vi "ME_acquire_22_HallSensor_LSchanB.vi"() -> ()   [LabVIEW 2015]
doc: "Use this template to build a producer/consumer design pattern. Use this template when you need to execute a process, such as data analysis, when a data source, such as a triggered acquisition, produces data at an uneven rate and you need to execute the process when the data becomes available."
uses:
  Mode.ctl
  oxford_driver/Oxford Drivers/BUSGEN.LLB/OxfordAddress.ctl
  <vilib>/Analysis/baseanly.llb/Mean (DBL).vi
  <vilib>/DAQmx/read.llb/DAQmx Read (Analog 1D DBL 1Chan NSamp).vi
  <vilib>/DAQmx/create/channels.llb/DAQmx Create Channel (AI-Voltage-Basic).vi
  <vilib>/DAQmx/configure/timing.llb/DAQmx Timing (Sample Clock).vi
  <vilib>/Utility/file.llb/Write Delimited Spreadsheet (DBL).vi
  <vilib>/DAQmx/miscellaneous.llb/DAQmx Fill In Error Info.vi
  <vilib>/express/express arith-compare/Formula/XNode/ExpressFormulaBlockNode.xnode
  <vilib>/Analysis/NI_AALBase.lvlib
panel:
  out "error out 2":errorcluster
  out "concatenated string":string
  out "error out":errorcluster
  out "B lag":cluster{dbl[], dbl[]}(graph)
  out "T array":dbl[](array[numeric])
  out "Averaged I(T)":dbl[][](array[numeric])
  in  "Averaged P(T)":dbl[][](array[numeric])
  out "remaining elements 2":T1(array[cluster])
  out "Actual mean":dbl format="%0.6f"
  in  "Averaged dt":dbl[][](array[numeric])
  in  "Averaged P(B)":dbl[][](array[numeric])
  out "deltaUaux":dbl
  out "Hall Resistance (Ohm)":dbl caption="Actual AuxV" step=0.1
  in  "Stop":bool
  out "SaveSweep":bool=TRUE
  out "Measurement File_dn":path
  out "Measurement File_up":path
  out "Measurement File_average":path
  out "Actual Polarization":dbl
  in  "Reset IB?":bool
  in  "First?":bool
  in  "Save Period":dbl=1.0
  out "Averaged I(B)":dbl[][](array[numeric])
  out "P(uC/mm^2)":dbl[](array[numeric])
  in  "Sweep":bool
  out "Offset array":dbl[](array[numeric])
  in  "stop 2":bool
  in  "dB":dbl=0.005
  out "Actual B Field (T)":dbl
  out "Actual Temperature (K)":dbl
  out "Actual Current (pA)":dbl
  in  "Tab Control":T2(tab)
  in  "Heater 2/1":bool
  in  "dt (K)":dbl=0.1
  in  "Max temperature (K)":dbl=20.0
  in  "Min Temperature (K)":dbl=4.5
  out "P(T)":cluster{"yi":dbl[], dbl[]}(graph)
  out "I(T)":cluster{dbl[], dbl[]}(graph)
  in  "Set temperature (K)":dbl=4.5
  in  "Temp Ramping Rate (K/min)":dbl=10.0
  in  "Heater Range":enum16{"Off", "Low", "Medium", "High"}(ring)
  in  "Heater On/Off":bool
  out "Setpoint Temperature (K)":dbl
  out "I(T) /Averaged/":cluster{"B array":dbl[], dbl[]}[](graph)
  out "P(T) /Averaged/":cluster{"B array":dbl[], dbl[]}[](graph)
  out "Up/Down 2":bool
  in  "Channel B/A":bool
  out "I(B) 3":cluster{dbl[], dbl[]}[](graph)
  out "I(B) /Averaged/":cluster{"B array":dbl[], dbl[]}[](graph)
  out "P(B) /Averaged/":cluster{"B array":dbl[], dbl[]}[](graph)
  out "P(B)":cluster{"yi":dbl[], dbl[]}(graph)
  in  "Set Field (T)":dbl
  in  "Go to Set":bool
  in  "Sweep Rate (T/min)":dbl=2.0 format="%.6f"
  in  "Field To Zero":bool
  out "Target Field":dbl
  in  "Min Field (T)":dbl
  in  "Max Field (T)":dbl=0.15
  in  "Threshold B (T)":dbl
  out "Up/Down":bool
  in  "Heater Range Array":i8[](array[numeric])=[1, 1, 1, 1, 1, 2, 2, 2, 2]
  in  "Magnetic Field array (T)":dbl[](array[numeric])=[0.025, 0.05, 0.075, 0.1, 0.125, 0.15, 0.175, 0.2, 0.225, 0.25, 0.275, 0.3]
  in  "T Sweep Rate Array":dbl[](array[numeric])=[10.0, 20.0]
  in  "Max count array":i32[](array[numeric])=[2, 1, 0, 0, 0, 9, 10, 11, 12]
  in  "secs to wait":dbl=180.0
  out "Wait (s)":dbl
  in  "Directory":string
  out "Finished":bool=TRUE
  out "Step Rate":bool
  out "New":bool=TRUE
  in  "Temperature Array":dbl[](array[numeric])=[4.5, 5.0, 6.0, 7.0, 8.0, 9.0, 10.0, 11.0, 12.0]
  in  "Sweep Rate Array":dbl[](array[numeric])=[2.0, 1.0, 0.5, 0.1, 0.05, 9.0, 10.0, 11.0, 12.0]
  in  "Record ALL":bool
  in  "Max Countl":i32
  out "i":i32
  out "j":i32
  out "Step Temp":bool
  in  "FileName":string
  in  "Measure Noise":bool
  in  "Cycles":i32
  in  "maximum value":dbl=10.0 format="%0.2f"
  in  "minimum value":dbl=-10.0 format="%0.2f"
  in  "physical channels":tag="Dev1/ai1"
  out "PSD (pA/Hz^1/2) Peaks Removed":cluster{"f0":dbl, "df":dbl, "magnitude":dbl[]}(graph)
  out "PSD (pA/Hz^1/2)":cluster{"f0":dbl, "df":dbl, "magnitude":dbl[]}(graph)
  out "Current (pA) Filtered":waveform(dbl)(graph)
  out "Current (pA)":dbl[](graph)
  in  "Samples per channel":i32=1000
  in  "Rate":dbl=1000.0 format="%0.2f"
  in  "Cut-Off Frequency":dbl=100.0 caption="Lower Cut-Off"
  in  "Filter On":bool
  in  "Keithley (IV conv) averaging":i32=10
  in  "Lock_in_Amplifier":refnum<visa-resource-name>="GPIB0::5::INSTR"
  out "Dc offset":dbl
  in  "Calibrate":bool
  in  "IV converter":refnum<visa-resource-name>="GPIB0::20::INSTR"
  in  "Magnetic Field":refnum<visa-resource-name>="GPIB0::19::INSTR"
  out "Time Lag":dbl=0.0500025749206543
  in  "Lake Shore":refnum<visa-resource-name>="GPIB0::11::INSTR"
  in  "Temp Refresh (s)":dbl=0.1
  in  "Sampling rate (Hz)":dbl=10.0
  in  "Gain (V/A)":dbl=1000000000.0
  in  "Sample area (mm^2)":dbl=1.0
  out "Calibration Curve":cluster{dbl[], "Best Linear Fit":dbl[]}[](graph)=[{[0.0, 0.005, 0.01, 0.015, 0.02, 0.025, 0.03, 0.035, 0.04, 0.045, 0.05, 0.055, 0.06, 0.065, 0.07, 0.075, 0.08, 0.085, 0.09, 0.095, 0.1, 0.105, 0.11, 0.115, 0.12, 0.125, 0.13, 0.135, 0.14, 0.145, 0.15, 0.155, 0.16, 0.165, 0.17, 0.175, 0.18, 0.185, 0.19, 0.195, 0.2, 0.205, 0.21, 0.215, 0.22, 0.225, 0.23, 0.235, 0.24, 0.245, 0.25, 0.255, 0.26, 0.265, 0.27, 0.275, 0.28, 0.285, 0.29, 0.295, 0.3, 0.305, 0.31, 0.315, 0.32, 0.325, 0.33, 0.335, 0.34, 0.345, 0.35, 0.355, 0.36, 0.365, 0.37, 0.375, 0.38, 0.385, 0.39, 0.395, 0.4, 0.405, 0.41, 0.415, 0.42, 0.425, 0.43, 0.435, 0.44, 0.445, 0.45, 0.455, 0.46, 0.465, 0.47, 0.475, 0.48, 0.485, 0.49, 0.495, 0.5], "Best Linear Fit"=[-1.7e-06, 1.18e-05, 3.66e-05, 6.17e-05, 9.39e-05, 0.000122, 0.0001511, 0.0001781, 0.0002061, 0.0002355, 0.0002616, 0.0002895, 0.0003184, 0.0003446, 0.0003689, 0.0003958, 0.0004207, 0.0004464, 0.0004684, 0.0004953, 0.0005218, 0.0005459, 0.0005692, 0.0005897, 0.0006131, 0.0006347, 0.0006589, 0.0006834, 0.0007035, 0.0007249, 0.0007465, 0.000765, 0.0007858, 0.0008103, 0.0008302, 0.0008467, 0.000868, 0.0008855, 0.0009079, 0.0009248, 0.0009452, 0.0009633, 0.0009828, 0.0009992, 0.0010189, 0.0010338, 0.001054, 0.0010692, 0.0010858, 0.0011036, 0.0011162, 0.0011356, 0.0011502, 0.0011643, 0.0011834, 0.0011985, 0.0012131, 0.0012277, 0.0012423, 0.0012571, 0.0012691, 0.0012827, 0.0012976, 0.001313, 0.0013264, 0.0013388, 0.0013518, 0.0013638, 0.0013782, 0.0013909, 0.0014035, 0.0014175, 0.0014295, 0.0014407, 0.0014538, 0.0014641, 0.0014752, 0.0014861, 0.0014978, 0.0015081, 0.0015203, 0.001532, 0.0015422, 0.0015526, 0.001563, 0.0015754, 0.0015844, 0.0015955, 0.0016056, 0.001614, 0.0016239, 0.0016342, 0.0016457, 0.0016542, 0.0016635, 0.001674, 0.001681, 0.0016886, 0.0016986, 0.0017063, 0.0017155]}, {[0.0, 0.005, 0.01, 0.015, 0.02, 0.025, 0.03, 0.035, 0.04, 0.045, 0.05, 0.055, 0.06, 0.065, 0.07, 0.075, 0.08, 0.085, 0.09, 0.095, 0.1, 0.105, 0.11, 0.115, 0.12, 0.125, 0.13, 0.135, 0.14, 0.145, 0.15, 0.155, 0.16, 0.165, 0.17, 0.175, 0.18, 0.185, 0.19, 0.195, 0.2, 0.205, 0.21, 0.215, 0.22, 0.225, 0.23, 0.235, 0.24, 0.245, 0.25, 0.255, 0.26, 0.265, 0.27, 0.275, 0.28, 0.285, 0.29, 0.295, 0.3, 0.305, 0.31, 0.315, 0.32, 0.325, 0.33, 0.335, 0.34, 0.345, 0.35, 0.355, 0.36, 0.365, 0.37, 0.375, 0.38, 0.385, 0.39, 0.395, 0.4, 0.405, 0.41, 0.415, 0.42, 0.425, 0.43, 0.435, 0.44, 0.445, 0.45, 0.455, 0.46, 0.465, 0.47, 0.475, 0.48, 0.485, 0.49, 0.495, 0.5], "Best Linear Fit"=[-1.7e-06, 1.18e-05, 3.66e-05, 6.17e-05, 9.39e-05, 0.000122, 0.0001511, 0.0001781, 0.0002061, 0.0002355, 0.0002616, 0.0002895, 0.0003184, 0.0003446, 0.0003689, 0.0003958, 0.0004207, 0.0004464, 0.0004684, 0.0004953, 0.0005218, 0.0005459, 0.0005692, 0.0005897, 0.0006131, 0.0006347, 0.0006589, 0.0006834, 0.0007035, 0.0007249, 0.0007465, 0.000765, 0.0007858, 0.0008103, 0.0008302, 0.0008467, 0.000868, 0.0008855, 0.0009079, 0.0009248, 0.0009452, 0.0009633, 0.0009828, 0.0009992, 0.0010189, 0.0010338, 0.001054, 0.0010692, 0.0010858, 0.0011036, 0.0011162, 0.0011356, 0.0011502, 0.0011643, 0.0011834, 0.0011985, 0.0012131, 0.0012277, 0.0012423, 0.0012571, 0.0012691, 0.0012827, 0.0012976, 0.001313, 0.0013264, 0.0013388, 0.0013518, 0.0013638, 0.0013782, 0.0013909, 0.0014035, 0.0014175, 0.0014295, 0.0014407, 0.0014538, 0.0014641, 0.0014752, 0.0014861, 0.0014978, 0.0015081, 0.0015203, 0.001532, 0.0015422, 0.0015526, 0.001563, 0.0015754, 0.0015844, 0.0015955, 0.0016056, 0.001614, 0.0016239, 0.0016342, 0.0016457, 0.0016542, 0.0016635, 0.001674, 0.001681, 0.0016886, 0.0016986, 0.0017063, 0.0017155]}]
  in  "Offset?":bool
  in  "Magnet":bool=TRUE
  in  "Ramp":bool=TRUE
  in  "DaQ":bool
  in  "Moving average":i8=10
  in  "Sample Rate":dbl=1000.0
  in  "Number of Samples":i32=100
  in  "Physical Channel":tag="kartya/ai0"
  in  "Min Voltage":dbl=-5.0
  in  "Max Voltage":dbl=5.0
  in  "Terminal Configuration":i32(ring)=-1 items=["default"=-1, "RSE"=10083, "NRSE"=10078, "Differential"=10106, "Pseudodifferential"=12529]
  out "Confirm":bool
  in  "Dwell Time (ms)":u32=1000
  out "Calibration Curve Data":dbl[][](array[numeric])=[[0.0, 0.005, 0.01, 0.015, 0.02, 0.025, 0.03, 0.035, 0.04, 0.045, 0.05, 0.055, 0.06, 0.065, 0.07, 0.075, 0.08, 0.085, 0.09, 0.095, 0.1, 0.105, 0.11, 0.115, 0.12, 0.125, 0.13, 0.135, 0.14, 0.145, 0.15, 0.155, 0.16, 0.165, 0.17, 0.175, 0.18, 0.185, 0.19, 0.195, 0.2, 0.205, 0.21, 0.215, 0.22, 0.225, 0.23, 0.235, 0.24, 0.245, 0.25, 0.255, 0.26, 0.265, 0.27, 0.275, 0.28, 0.285, 0.29, 0.295, 0.3, 0.305, 0.31, 0.315, 0.32, 0.325, 0.33, 0.335, 0.34, 0.345, 0.35, 0.355, 0.36, 0.365, 0.37, 0.375, 0.38, 0.385, 0.39, 0.395, 0.4, 0.405, 0.41, 0.415, 0.42, 0.425, 0.43, 0.435, 0.44, 0.445, 0.45, 0.455, 0.46, 0.465, 0.47, 0.475, 0.48, 0.485, 0.49, 0.495, 0.5], [-1.7e-06, 1.18e-05, 3.66e-05, 6.17e-05, 9.39e-05, 0.000122, 0.0001511, 0.0001781, 0.0002061, 0.0002355, 0.0002616, 0.0002895, 0.0003184, 0.0003446, 0.0003689, 0.0003958, 0.0004207, 0.0004464, 0.0004684, 0.0004953, 0.0005218, 0.0005459, 0.0005692, 0.0005897, 0.0006131, 0.0006347, 0.0006589, 0.0006834, 0.0007035, 0.0007249, 0.0007465, 0.000765, 0.0007858, 0.0008103, 0.0008302, 0.0008467, 0.000868, 0.0008855, 0.0009079, 0.0009248, 0.0009452, 0.0009633, 0.0009828, 0.0009992, 0.0010189, 0.0010338, 0.001054, 0.0010692, 0.0010858, 0.0011036, 0.0011162, 0.0011356, 0.0011502, 0.0011643, 0.0011834, 0.0011985, 0.0012131, 0.0012277, 0.0012423, 0.0012571, 0.0012691, 0.0012827, 0.0012976, 0.001313, 0.0013264, 0.0013388, 0.0013518, 0.0013638, 0.0013782, 0.0013909, 0.0014035, 0.0014175, 0.0014295, 0.0014407, 0.0014538, 0.0014641, 0.0014752, 0.0014861, 0.0014978, 0.0015081, 0.0015203, 0.001532, 0.0015422, 0.0015526, 0.001563, 0.0015754, 0.0015844, 0.0015955, 0.0016056, 0.001614, 0.0016239, 0.0016342, 0.0016457, 0.0016542, 0.0016635, 0.001674, 0.001681, 0.0016886, 0.0016986, 0.0017063, 0.0017155]]
  in  "Start Field":dbl
  in  "Max Field":dbl=0.5 format="%#_13g"
  in  "Reoffset?":bool
  in  "Temp/Magnetic Field":bool
  out "index":i8
  out "Read?":bool
  out "Magnetic Field (T)":dbl[](array[numeric])
  out "Reset":bool
  out "Measured Current (pA)":dbl[](array[numeric])
  out "Elapsed Time (s)":dbl[](array[numeric])
  out "Start time":timestamp
  in  "Enum":T3=enum."Process"
  out "B array":dbl[](array[numeric])
  in  "dB (T)":dbl=0.0025
  in  "Counter":i8
  out "L magnet (H)":dbl
  out "R magnet (mOhm)":dbl
  out "Actual Current (R0)":dbl
  out "Nominal Field (T)":dbl
  out "Temperature array":dbl[](array[numeric])
  in  "New Measurement File":bool
  out "Measurement File":path
  out "refnum out":refnum<file>
  in  "Measuring":bool
  in  "Measure /Pause":bool
  in  "stop":bool
  # "DeltaForce"
  # "Discrete"
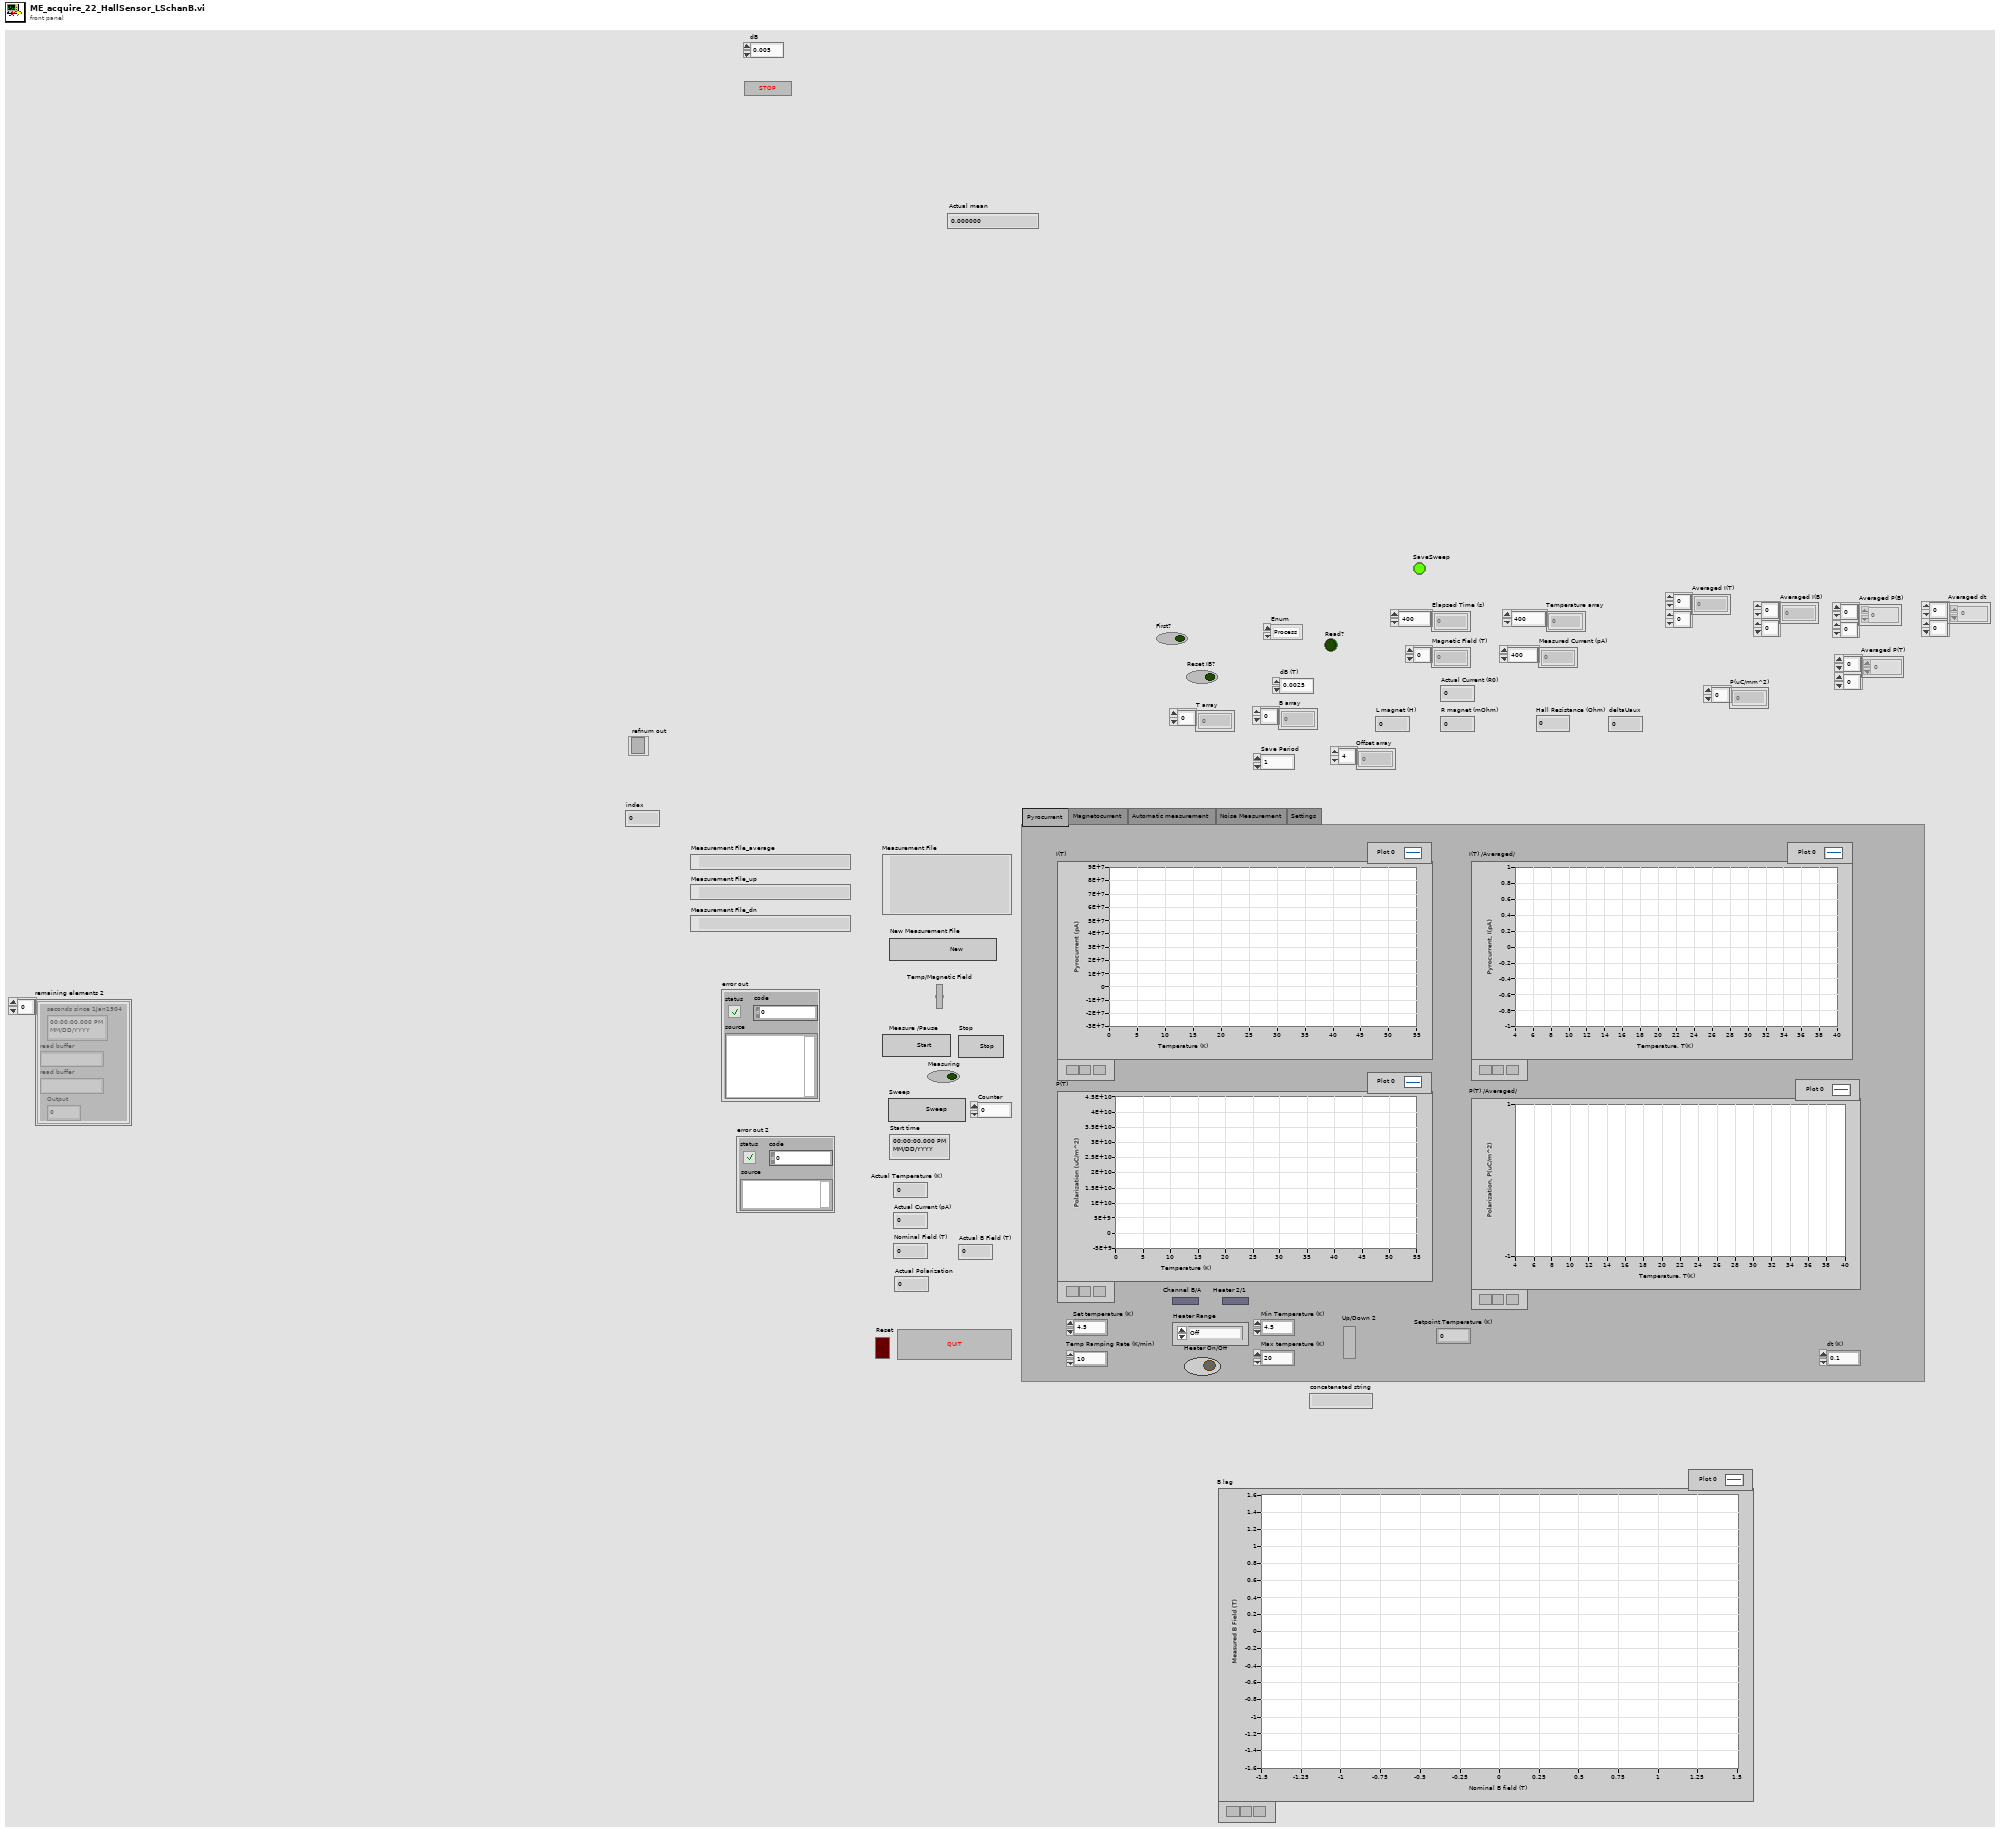
[diagram p1: front panel]
types:
  T1 = cluster{"seconds since 1Jan1904":timestamp, "read buffer":string, "read buffer":string, "Output":dbl}[]
  T2 = enum32{"Pyrocurrent", "Magnetocurrent", "Automatic measurement", "Noise Measurement", "Settings"}
  T3 = typedef "Mode.ctl" = enum16{"Offset", "Process", "Sweep", "StepOxford", "StepDelta", "Plot", "Save", "New", "Return", ""}
  T4 = cluster{"seconds since 1Jan1904":timestamp, "read buffer":string, "read buffer":string, "Output":dbl}
  T5 = enum16{"open", "replace", "create", "open or create", "replace or create", "replace or create with confirmation"}
  T6 = typedef "OxfordAddress.ctl" = cluster{"Com Port":i32, "ISOBUS Address":i32, "GPIB Address":i16, "Communication":enum16{"RS232", "ISOBUS", "GPIB", "Gateway"}}
  T7 = cluster{"B array":dbl[], "Averaged P(B) Out":dbl[]}
  T8 = cluster{"B array":dbl[], "BaselineSubtracted I(B)":dbl[]}
  T9 = cluster{"B array":dbl[], "Averaged P(B) Out":dbl[]}[]
  T10 = cluster{"B array":dbl[], "BaselineSubtracted I(B)":dbl[]}[]
  T11 = cluster{"T array":dbl[], "Averaged P(T) Out":dbl[]}
  T12 = cluster{"T array":dbl[], "Averaged I(B) out":dbl[]}
  T13 = cluster{"T array":dbl[], "Averaged P(T) Out":dbl[]}[]
  T14 = cluster{"T array":dbl[], "Averaged I(B) out":dbl[]}[]
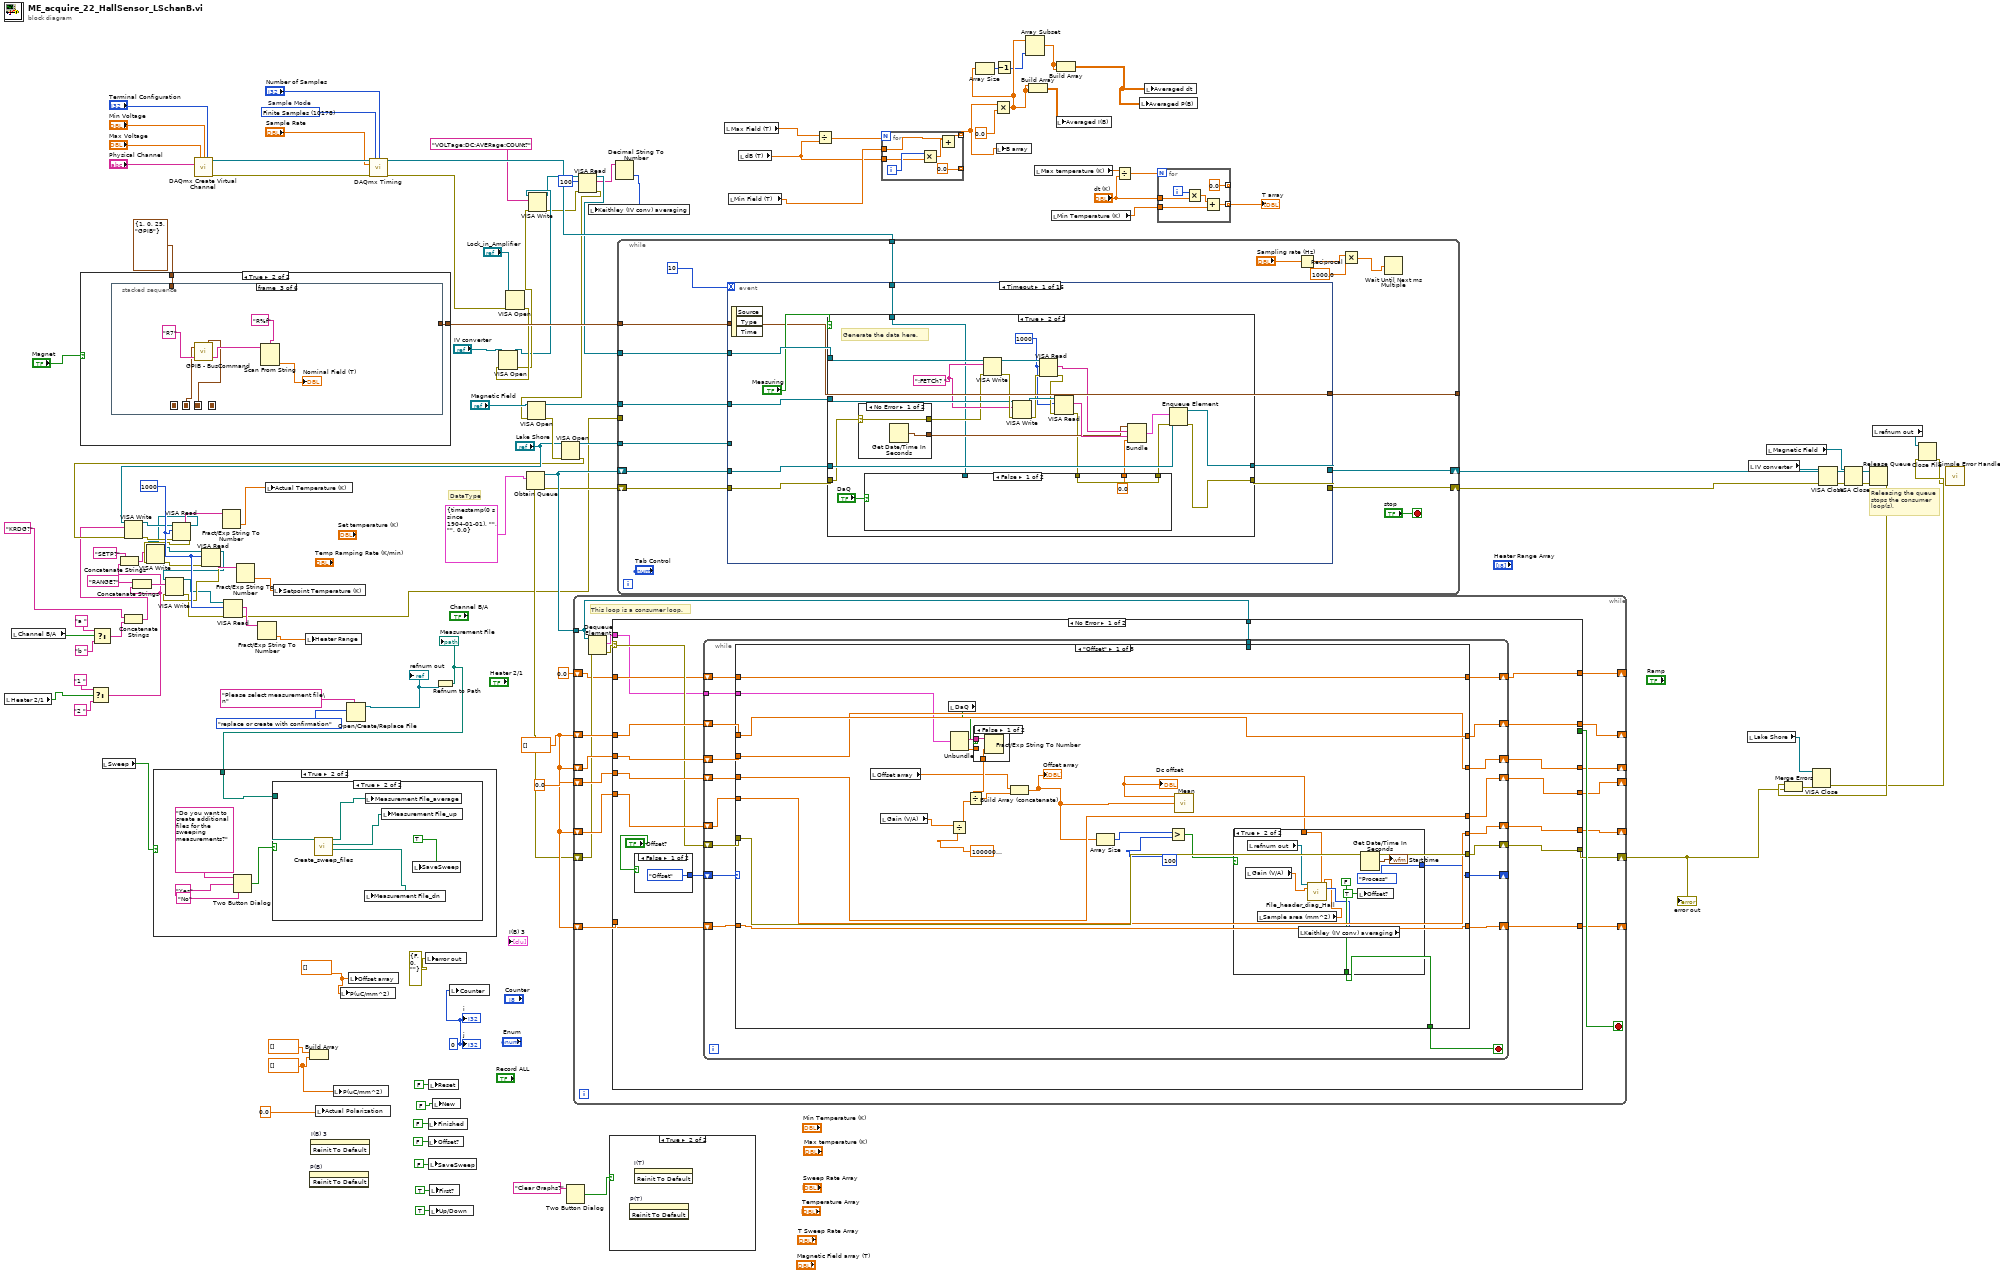
[diagram p0: block diagram]
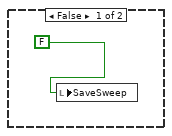
[diagram p4: hidden frame]
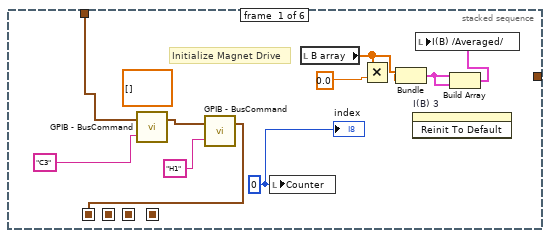
[diagram p6: hidden frame]
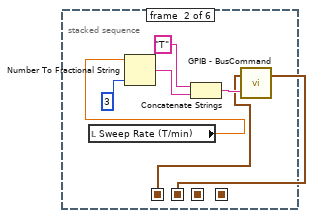
[diagram p7: hidden frame]
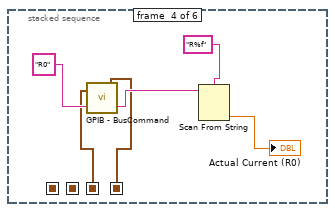
[diagram p8: hidden frame]
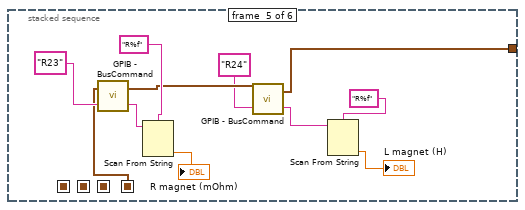
[diagram p9: hidden frame]
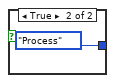
[diagram p11: hidden frame]
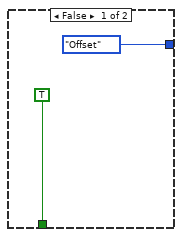
[diagram p13: hidden frame]
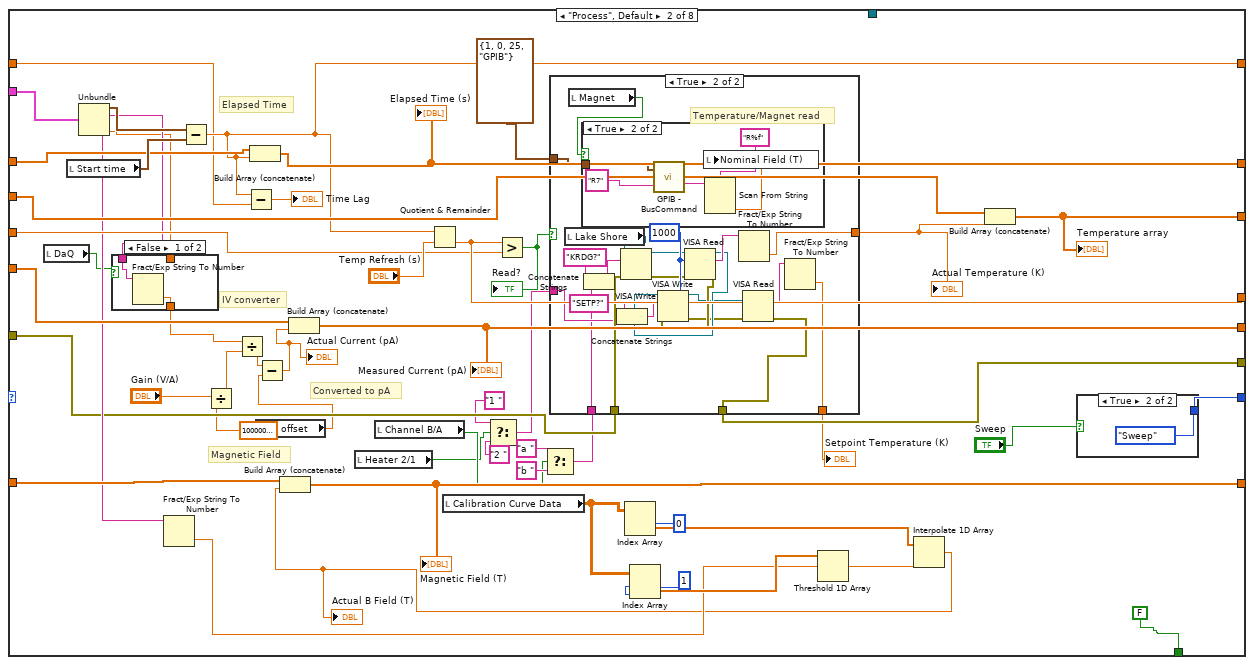
[diagram p14: hidden frame]
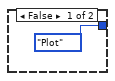
[diagram p16: hidden frame]
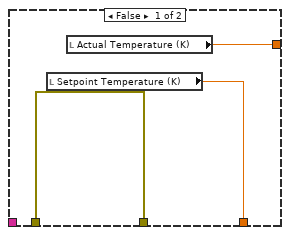
[diagram p17: hidden frame]
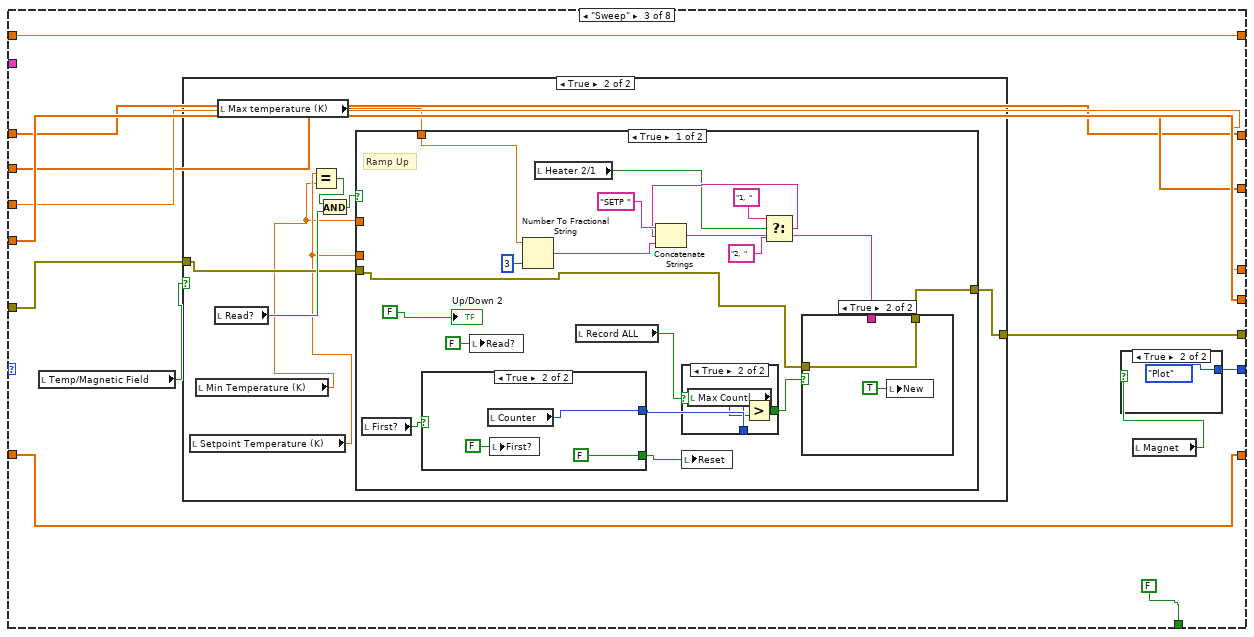
[diagram p19: hidden frame]
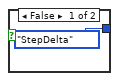
[diagram p20: hidden frame]
diagram:
  w43 = 10178 items=["Finite Samples"=10178, "Continuous Samples"=10123, "Hardware Timed Single Point"=12522]  # Sample Mode
  w70 = u32 1000 ("byte count")
  w78 = 0 ("j")
  w75 = dbl[] []
  w93 = dbl[] []
  w99 = dbl[] []
  # "DataType"
  # "Releasing the queue stops the consumer loop(s)."
  n1 = local read "Heater 2/1"() -> (w1:bool)
  n2 = local read "Channel B/A"() -> (w3:bool)
  n3 = case shown="True" "Magnet" {
    tunnel: T6 {"Com Port"=1, "ISOBUS Address"=0, "GPIB Address"=25, "Communication"=enum."GPIB"} ("Address") -> [w122 w124]
    tunnel: [w122 w123] -> w105
    frame False {
    }
    frame True {
      n4 = stacked-sequence {
        seq-local: [w132 _ _ _ _ _] -> [_ w137 _ _ _ _]
        seq-local: [_ w136 _ _ _ _] -> [_ _ w144 _ _ _]
        seq-local: [_ _ w143 _ _ _] -> [_ _ _ w150 _ _]
        seq-local: [_ _ _ w149 _ _] -> [_ _ _ _ w161 _]
        tunnel: w124 -> [w134 _ _ _ _ _]
        tunnel: [_ _ _ _ w159 _] -> w123
        frame #0 {
          (unwired) dbl[][] []
          w130 = i8 0 ("Counter")
          # "Initialize Magnet Drive"
          n5 = call "GPIB - BusCommand.vi"("Command"="C3", "Address"=w134) -> ("Address(thru)"=w133:T6)  [unwired: 1 out]
          n6 = call "GPIB - BusCommand.vi"("Command"="H1", "Address"=w133) -> ("Address(thru)"=w132:T6)  [unwired: 1 out]
          n7 = local write "Counter"(w130) -> ()
          n8 = local read "B array"() -> (w128:dbl[])
          n9 = Multiply(x=w128, y=0.0) -> (x*y=w127:dbl[])
          n10 = Bundle("B array"=w128, w127) -> (w126:cluster{"B array":dbl[], dbl[]})  [unwired: 1 in]
          n11 = invoke on="I(B) 3" class="XYGraph (strict)" method="Reinit To Default"() -> ()  [unwired: 3 in, 3 out]
          n12 = Build Array(w126, w126) -> (w125:cluster{"B array":dbl[], dbl[]}[])
          n13 = local write "I(B) /Averaged/"(w125) -> ()
          "index" <- w130
        }
        frame #1 {
          n14 = local read "Sweep Rate (T/min)"() -> (w138:dbl)
          n15 = Number To Fractional String(number=w138, precision (6)=i16 3) -> (F-format string=w140:string)  [unwired: 2 in]
          n16 = Concatenate Strings("T" ("format string"), w140) -> (w139:string)
          n17 = call "GPIB - BusCommand.vi"("Command"=w139, "Address"=w137) -> ("Address(thru)"=w136:T6)  [unwired: 1 out]
        }
        frame #2 {
          n18 = call "GPIB - BusCommand.vi"("Command"="R7" ("format string"), "Address"=w144) -> ("Reply"=w148:string, "Address(thru)"=w143:T6)
          n19 = Scan From String(format string="R%f" ("remaining string"), input string=w148) -> (output 1=→"Nominal Field (T)":dbl)  [unwired: 3 in, 3 out]
        }
        frame #3 {
          n20 = call "GPIB - BusCommand.vi"("Command"="R0" ("format string"), "Address"=w150) -> ("Reply"=w154:string, "Address(thru)"=w149:T6)
          n21 = Scan From String(format string="R%f" ("remaining string"), input string=w154) -> (output 1=→"Actual Current (R0)":dbl)  [unwired: 3 in, 3 out]
        }
        frame #4 {
          n22 = call "GPIB - BusCommand.vi"("Command"="R23" ("format string"), "Address"=w161) -> ("Reply"=w165:string, "Address(thru)"=w160:T6)
          n23 = Scan From String(format string="R%f" ("remaining string"), input string=w165) -> (output 1=→"R magnet (mOhm)":dbl)  [unwired: 3 in, 3 out]
          n24 = call "GPIB - BusCommand.vi"("Command"="R24" ("format string"), "Address"=w160) -> ("Reply"=w157:string, "Address(thru)"=w159:T6)
          n25 = Scan From String(format string="R%f" ("remaining string"), input string=w157) -> (output 1=→"L magnet (H)":dbl)  [unwired: 3 in, 3 out]
        }
        frame #5 {
        }
      }
    }
  }
  n26 = Select(t="1 " ("write buffer"), s=w1, f="2 " ("write buffer")) -> (s? t:f=w2:string)
  n27 = Select(t="a " ("write buffer"), s=w3, f="b " ("write buffer")) -> (s? t:f=w9:string)
  n28 = local read "Sweep"() -> (w83:bool)
  n29 = Concatenate Strings("SETP?" ("write buffer"), w2) -> (w11:string)
  n30 = Concatenate Strings("KRDG?" ("write buffer"), w9) -> (w13:string)
  n31 = Concatenate Strings("RANGE?" ("write buffer"), w2) -> (w8:string)
  n32 = call-poly <vilib>:"DAQmx Create Virtual Channel.vi"("maximum value"="Max Voltage", "minimum value"="Min Voltage", "input terminal configuration"="Terminal Configuration", "physical channels"="Physical Channel") -> ("task out"=w41:refnum<k21>, "error out"=w42:errorcluster)  [unwired: 10 in]
  n33 = Build Array(dbl[] [], w75) -> ()  [unwired: 1 out]
  n34 = invoke on="P(B)" class="XYGraph (strict)" method="Reinit To Default"() -> ()  [unwired: 3 in, 3 out]
  n35 = invoke on="I(B) 3" class="XYGraph (strict)" method="Reinit To Default"() -> ()  [unwired: 3 in, 3 out]
  n36 = local write "Actual Polarization"(0.0 ("Actual Polarization")) -> ()
  n37 = local write "P(uC/mm^2)"(w75) -> ()
  n38 = local write "P(uC/mm^2)"(w93) -> ()
  n39 = Open/Create/Replace File(prompt="Please select measurement file\n", operation (0:open)=T5."replace or create with confirmation") -> (refnum out=w102:refnum<file>)  [unwired: 4 in, 2 out]
  "refnum out" <- w102
  n40 = local write "Offset array"(w93) -> ()
  n41 = call-poly <vilib>:"DAQmx Timing.vi"("task/channels in"=w41, "sample mode"=w43, "samples per channel"="Number of Samples", "rate"="Sample Rate", "error in"=w42) -> ("task out"=w33:refnum<k21>, "error out"=w34:errorcluster)  [unwired: 9 in]
  n42 = local write "error out"(errorcluster {"status"=FALSE, "code"=0, "source"=""} ("error constant")) -> ()
  n43 = local write "Finished"(FALSE ("Finished")) -> ()
  n44 = local write "Offset?"(FALSE ("Offset?")) -> ()
  n45 = local write "Reset"(FALSE ("Reset")) -> ()
  n46 = local write "SaveSweep"(FALSE ("SaveSweep")) -> ()
  n47 = local write "First?"(TRUE ("First?")) -> ()
  n48 = local write "Up/Down"(TRUE ("Up/Down")) -> ()
  n49 = local write "New"(FALSE ("New")) -> ()
  n50 = Refnum to Path(1:w102) -> (0:w82:path)
  "Measurement File" <- w82
  n51 = case shown="True" w83 {
    tunnel: w82 -> [_ w166]
    frame False {
    }
    frame True {
      n52 = Two Button Dialog(message="Do you want to create additional files for the sweeping measurements?" ("string"), 1:"No" ("F button name (\"Cancel\")"), 2:"Yes" ("T button name (\"OK\")")) -> (T button?=w168:bool)
      n53 = case shown="True" w168 {
        tunnel: w166 -> [_ w176]
        frame False {
          n54 = local write "SaveSweep"(FALSE ("SaveSweep")) -> ()
        }
        frame True {
          n55 = call "Create_sweep_files.vi"("Measurement File"=w176) -> ("Path 3"=w173:path, "Path 2"=w174:path, "Path"=w175:path)  [unwired: 8 in]
          n56 = local write "Measurement File_dn"(w173) -> ()
          n57 = local write "Measurement File_average"(w175) -> ()
          n58 = local write "Measurement File_up"(w174) -> ()
          n59 = local write "SaveSweep"(TRUE) -> ()
        }
      }
    }
  }
  n60 = local write "Counter"(w78) -> ()
  n61 = VISA Open(error in (no error)=w34, VISA resource name="Lock_in_Amplifier") -> (error out=w53:errorcluster)  [unwired: 3 in, 1 out]
  n62 = VISA Open(error in (no error)=w53, VISA resource name="IV converter") -> (VISA resource name=w30:refnum<visa-resource-name>, error out=w31:errorcluster)  [unwired: 3 in]
  n63 = Obtain Queue(element data type=T4 {"seconds since 1Jan1904"=timestamp(0 s since 1904-01-01), "read buffer"="", "read buffer"="", "Output"=0.0} ("output cluster")) -> (queue out=w121:refnum<queue>, error out=w97:errorcluster)  [unwired: 4 in, 1 out]
  n64 = VISA Write(VISA resource name=w30, write buffer="VOLTage:DC:AVERage:COUNt?", error in (no error)=w31) -> (VISA resource name out=w26:refnum<visa-resource-name>, error out=w28:errorcluster)  [unwired: 1 out]
  n65 = Two Button Dialog(message="Clear Graphs?") -> (T button?=w77:bool)  [unwired: 2 in]
  n66 = while {
    tunnel: w121 -> [w177]
    shift-right: [w190] -> _
    shift-left: w99 -> [w189]
    shift-right: [w188] -> _
    shift-left: w99 -> [w187]
    shift-right: [w186] -> _
    shift-left: w99 -> [w185]
    shift-right: [w184] -> _
    shift-left: 0.0 -> [w183]
    shift-right: [w182] -> _
    shift-left: w99 -> [w181]
    shift-right: [w191] -> w7
    shift-left: w97 -> [w180]
    shift-right: [w179] -> _
    shift-left: 0.0 -> [w178]
    stop <- w192 stop-if-true
    # "This loop is a consumer loop."
    n67 = Dequeue Element(queue=w177, error in (no error)=w180) -> (element=w193:T4, error out=w194:errorcluster)  [unwired: 1 in, 2 out]
    n68 = case shown="No Error" w194 {
      selector: w194 -> [w201 w1008]
      tunnel: w193 -> [w195 _]
      tunnel: [_ TRUE] -> w192
      tunnel: [w200 w1008] -> w191
      tunnel: [w211 w1007] -> w190
      tunnel: w189 -> [w210 w1007]
      tunnel: [w209 w1004] -> w188
      tunnel: w187 -> [w208 w1004]
      tunnel: [w207 w1003] -> w186
      tunnel: w185 -> [w206 w1003]
      tunnel: [w205 w1005] -> w184
      tunnel: w183 -> [w204 w1005]
      tunnel: [w203 w1006] -> w182
      tunnel: w181 -> [w202 w1006]
      tunnel: [w199 w1002] -> w179
      tunnel: w178 -> [w198 w1002]
      tunnel: w177 -> [w196 _]
      frame No Error {
        n69 = case shown="False" "Offset?" {
          tunnel: [Mode."Offset" ("Enum") Mode."Process" ("Enum")] -> w212
          frame False {
          }
          frame True {
          }
        }
        n70 = while {
          shift-right: [w221] -> _
          shift-left: w212 -> [w233]
          tunnel: w195 -> [w232]
          shift-right: [w231] -> w211
          shift-left: w210 -> [w230]
          shift-right: [w223] -> w203
          shift-left: w202 -> [w222]
          shift-right: [w225] -> w205
          shift-left: w204 -> [w224]
          shift-right: [w229] -> w209
          shift-left: w208 -> [w228]
          shift-right: [w219] -> w200
          shift-left: w201 -> [w220]
          shift-right: [w227] -> w207
          shift-left: w206 -> [w226]
          shift-right: [w217] -> w199
          shift-left: w198 -> [w216]
          tunnel: w196 -> [w215]
          stop <- w218 stop-if-true
          n71 = case shown="\"Offset\"" w233 {
            selector: w233 -> [_ _ _ _ _ _ _ w995]
            tunnel: w232 -> [w251 w322 _ _ _ _ _ _]
            tunnel: [w257 w319 w364 w506 w562 w635 w749 w1000] -> w231
            tunnel: w230 -> [w257 w314 w364 w506 w562 w631 w749 w1000]
            tunnel: [w252 w318 w367 w503 w564 w637 w747 w997] -> w229
            tunnel: w228 -> [w252 w317 w367 w503 w564 w632 w747 w997]
            tunnel: [w253 w316 w369 w501 w559 w638 w745 w994] -> w227
            tunnel: w226 -> [w253 w315 w369 w501 w559 w633 w745 w994]
            tunnel: [w255 w313 w366 w504 w560 w641 0.0 w998] -> w225
            tunnel: w224 -> [w255 w312 w366 w504 w560 w641 _ w998]
            tunnel: [w256 w309 w365 w505 w561 w636 w748 w999] -> w223
            tunnel: w222 -> [w256 w310 w365 w505 w561 w634 w748 w999]
            tunnel: [w240 w307 w362 Mode."Plot" ("Enum") Mode."Save" ("Enum") w642 Mode."Return" ("Enum") w995] -> w221
            tunnel: w220 -> [w254 w305 w371 w498 w567 w640 w741 w996]
            tunnel: [w254 w304 w370 w497 w567 w640 w740 w996] -> w219
            tunnel: [w236 FALSE FALSE FALSE FALSE w629 TRUE TRUE] -> w218
            tunnel: [w239 w301 w363 w499 w563 w639 0.0 w1001] -> w217
            tunnel: w216 -> [w239 w300 w363 w499 w563 w639 _ w1001]
            tunnel: w215 -> [_ _ _ _ _ _ w739 _]
            frame "Offset" {
              n72 = local read "Offset array"() -> (w245:dbl[])
              n73 = local read "Gain (V/A)"() -> (w249:dbl)
              n74 = local read "DaQ"() -> (w235:bool)
              n75 = Unbundle(w251) -> ("read buffer"=w238:string, "Output"=w234:dbl)  [unwired: 2 out]
              n76 = Divide(x=w249, y=1000000000000.0) -> (x/y=w247:dbl)
              n77 = case shown="False" w235 {
                tunnel: [w259 w260] -> w250
                tunnel: w238 -> [w258 _]
                tunnel: w234 -> [_ w260]
                frame False {
                  n78 = Fract/Exp String To Number(string=w258) -> (number=w259:dbl)  [unwired: 3 in, 1 out]
                }
                frame True {
                }
              }
              n79 = Divide(x=w250, y=w247) -> (x/y=w246:dbl)
              n80 = Build Array (concatenate)(w245, w246) -> (w241:dbl[])
              "Offset array" <- w241
              n81 = Array Size(array=w241) -> (size(s)=w244:i32)
              n82 = Greater?(x=w244, y=100) -> (0:w242:bool)
              n83 = call-poly <vilib>:"Mean.vi"("X"=w241) -> ("mean"=w237:dbl)  [unwired: 1 out]
              "Dc offset" <- w237
              n84 = case shown="True" w242 {
                tunnel: [Mode."Offset" ("Enum") Mode."Process" ("Enum")] -> w240
                tunnel: w237 -> [_ w267]
                tunnel: [TRUE FALSE] -> w236
                frame False {
                }
                frame True {
                  n85 = local read "Gain (V/A)"() -> (w268:dbl)
                  n86 = local read "refnum out"() -> (w269:refnum<file>)
                  n87 = local read "Sample area (mm^2)"() -> (w263:dbl)
                  n88 = local read "Keithley (IV conv) averaging"() -> (w264:i32)
                  n89 = call "File_header_diag_Hall.vi"("Byte Stream File in"=w269, "OFFSET"=w267, "Sample area"=w263, "Gain"=w268, "Averaging"=w264) -> ()  [unwired: 11 in]
                  n90 = local write "Offset?"(TRUE ("Offset?")) -> ()
                  n91 = Get Date/Time In Seconds() -> (seconds since 1Jan1904=→"Start time":timestamp)
                }
              }
            }
            frame "Process", Default {
              # "Converted to pA"
              # "Magnetic Field"
              # "IV converter"
              # "Elapsed Time"
              n92 = local read "DaQ"() -> (w290:bool)
              n93 = local read "Start time"() -> (w320:timestamp)
              n94 = Unbundle(w322) -> ("seconds since 1Jan1904"=w321:timestamp, "read buffer"=w291:string, "read buffer"=w306:string, "Output"=w288:dbl)
              n95 = case shown="False" w290 {
                tunnel: w291 -> [w326 _]
                tunnel: [w325 w327] -> w289
                tunnel: w288 -> [_ w327]
                frame False {
                  n96 = Fract/Exp String To Number(string=w326) -> (number=w325:dbl)  [unwired: 3 in, 1 out]
                }
                frame True {
                }
              }
              n97 = Fract/Exp String To Number(string=w306) -> (number=w283:dbl)  [unwired: 3 in, 1 out]
              n98 = Subtract(x=w321, y=w320) -> (x-y=w301:dbl)
              n99 = Divide(x="Gain (V/A)", y=1000000000000.0) -> (x/y=w299:dbl)
              n100 = Divide(x=w289, y=w299) -> (x/y=w296:dbl)
              n101 = Subtract(x=w301, y=w300) -> (x-y=→"Time Lag":dbl)
              n102 = Build Array (concatenate)(w314, w301) -> (w319:dbl[])
              "Elapsed Time (s)" <- w319
              n103 = local read "Dc offset"() -> (w294:dbl)
              n104 = Subtract(x=w296, y=w294) -> (x-y=w295:dbl)
              "Actual Current (pA)" <- w295
              n105 = Build Array (concatenate)(w317, w295) -> (w318:dbl[])
              "Measured Current (pA)" <- w318
              n106 = local read "Heater 2/1"() -> (w272:bool)
              n107 = local read "Channel B/A"() -> (w275:bool)
              n108 = Quotient & Remainder(x=w301, y="Temp Refresh (s)") -> (floor(x/y)=w313:dbl)  [unwired: 1 out]
              n109 = local read "Calibration Curve Data"() -> (w285:dbl[][])
              n110 = Select(t="1 " ("write buffer"), s=w272, f="2 " ("write buffer")) -> (s? t:f=w278:string)
              n111 = Greater?(x=w313, y=w312) -> (0:w311:bool)
              "Read?" <- w311
              n112 = Select(t="a " ("write buffer"), s=w275, f="b " ("write buffer")) -> (s? t:f=w274:string)
              n113 = case shown="True" w311 {
                tunnel: [w331 w353] -> w308
                tunnel: w305 -> [w332 w352]
                tunnel: [w332 w334] -> w304
                tunnel: T6 {"Com Port"=1, "ISOBUS Address"=0, "GPIB Address"=25, "Communication"=enum."GPIB"} ("Address") -> [_ w351]
                tunnel: [w330 w348] -> w292
                tunnel: w278 -> [_ w336]
                tunnel: w274 -> [_ w333]
                frame False {
                  n114 = local read "Setpoint Temperature (K)"() -> (w330:dbl)
                  n115 = local read "Actual Temperature (K)"() -> (w331:dbl)
                }
                frame True {
                  w349 = u32 1000 ("byte count")
                  # "Temperature/Magnet read"
                  n116 = local read "Lake Shore"() -> (w350:refnum<visa-resource-name>)
                  n117 = local read "Magnet"() -> (w340:bool)
                  n118 = case shown="True" w340 {
                    tunnel: w351 -> [_ w356]
                    frame False {
                    }
                    frame True {
                      n119 = call "GPIB - BusCommand.vi"("Command"="R7" ("format string"), "Address"=w356) -> ("Reply"=w357:string)  [unwired: 1 out]
                      n120 = Scan From String(format string="R%f" ("remaining string"), input string=w357) -> (output 1=w355:dbl)  [unwired: 3 in, 3 out]
                      n121 = local write "Nominal Field (T)"(w355) -> ()
                    }
                  }
                  n122 = Concatenate Strings("KRDG?" ("write buffer"), w333) -> (w335:string)
                  n123 = Concatenate Strings("SETP?" ("write buffer"), w336) -> (w337:string)
                  n124 = VISA Write(VISA resource name=w350, write buffer=w335, error in (no error)=w352) -> (VISA resource name out=w347:refnum<visa-resource-name>, error out=w345:errorcluster)  [unwired: 1 out]
                  n125 = VISA Read(VISA resource name=w347, byte count=w349, error in (no error)=w345) -> (VISA resource name out=w346:refnum<visa-resource-name>, read buffer=w354:string, error out=w344:errorcluster)  [unwired: 1 out]
                  n126 = VISA Write(VISA resource name=w346, write buffer=w337, error in (no error)=w344) -> (VISA resource name out=w342:refnum<visa-resource-name>, error out=w343:errorcluster)  [unwired: 1 out]
                  n127 = Fract/Exp String To Number(string=w354) -> (number=w353:dbl)  [unwired: 3 in, 1 out]
                  n128 = VISA Read(VISA resource name=w342, byte count=w349, error in (no error)=w343) -> (read buffer=w341:string, error out=w334:errorcluster)  [unwired: 2 out]
                  n129 = Fract/Exp String To Number(string=w341) -> (number=w348:dbl)  [unwired: 3 in, 1 out]
                }
              }
              "Actual Temperature (K)" <- w308
              "Setpoint Temperature (K)" <- w292
              n130 = Index Array(array=w285, index (row)=0) -> (element=w281:dbl[])  [unwired: 1 in]
              n131 = Index Array(array=w285, index (row)=1 ("index (col)")) -> (element=w284:dbl[])  [unwired: 1 in]
              n132 = Threshold 1D Array(2:w283, 3:w284) -> (0:w282:dbl)  [unwired: 1 in]
              n133 = Interpolate 1D Array(1:w282, 2:w281) -> (0:w273:dbl)
              "Actual B Field (T)" <- w273
              n134 = Build Array (concatenate)(w315, w273) -> (w316:dbl[])
              "Magnetic Field (T)" <- w316
              n135 = Build Array (concatenate)(w310, w308) -> (w309:dbl[])
              "Temperature array" <- w309
              n136 = case shown="True" "Sweep" {
                tunnel: [Mode."Plot" ("Enum") Mode."Sweep" ("Enum")] -> w307
                frame False {
                }
                frame True {
                }
              }
            }
            frame "Sweep" {
              n137 = local read "Temp/Magnetic Field"() -> (w361:bool)
              n138 = case shown="True" w361 {
                tunnel: w371 -> [w380 w437]
                tunnel: [w379 w436] -> w370
                frame False {
                  n139 = local read "Nominal Field (T)"() -> (w375:dbl)
                  n140 = local read "Min Field (T)"() -> (w374:dbl)
                  n141 = local read "Max Field (T)"() -> (w381:dbl)
                  n142 = local read "Read?"() -> (w378:bool)
                  n143 = Greater Or Equal?(x=w374, y=w375) -> (x >= y?=w377:bool)
                  n144 = Compound Arithmetic op=AND(w377, w378) -> (w376:bool)
                  n145 = case shown="True" w376 {
                    tunnel: [w384 w420] -> w379
                    tunnel: w381 -> [w382 w419]
                    tunnel: w374 -> [_ w418]
                    tunnel: w375 -> [_ w416]
                    tunnel: w380 -> [w385 w415]
                    frame True {
                      # "Ramp Up"
                      n146 = case shown="False" "First?" {
                        tunnel: [TRUE ("Save") FALSE ("Save")] -> w388
                        tunnel: [w407 w411] -> w387
                        frame False {
                          n147 = local read "Counter"() -> (w410:i8)
                          n148 = local write "Actual Polarization"(0.0 ("Actual Polarization")) -> ()
                          n149 = Increment(x=w410) -> (x+1=w407:i8)
                          n150 = local write "Counter"(w407) -> ()
                        }
                        frame True {
                          n151 = local read "Counter"() -> (w411:i8)
                          n152 = local write "First?"(FALSE ("First?")) -> ()
                        }
                      }
                      "Reset" <- w388
                      n153 = local write "Read?"(FALSE ("Read?")) -> ()
                      n154 = local read "Record ALL"() -> (w383:bool)
                      n155 = case shown="True" w383 {
                        tunnel: w387 -> [_ w395]
                        tunnel: [FALSE w393] -> w386
                        frame False {
                        }
                        frame True {
                          n156 = Greater?(x=w395, y="Max Countl") -> (0:w393:bool)
                        }
                      }
                      n157 = case shown="False" w386 {
                        tunnel: w385 -> [w399 w406]
                        tunnel: [w398 w406] -> w384
                        tunnel: w382 -> [w397 _]
                        frame False {
                          n158 = local read "Magnet"() -> (w396:bool)
                          n159 = case shown="True" w396 {
                            tunnel: w399 -> [w400 w403]
                            tunnel: [w400 w402] -> w398
                            tunnel: w397 -> [_ w401]
                            frame False {
                            }
                            frame True {
                              n160 = call "Set_B.vi"("error in (no error)"=w403, "address string"="25", "Set Field (T)"=w401) -> ("error out"=w402:errorcluster)  [unwired: 8 in]
                            }
                          }
                          "Target Field" <- w397
                        }
                        frame True {
                          "New" <- TRUE
                        }
                      }
                      "Up/Down" <- FALSE ("Up/Down")
                    }
                    frame False {
                      n161 = Less Or Equal?(x=w419, y=w416) -> (x <= y?=w417:bool)
                      n162 = case shown="False" w417 {
                        tunnel: [w421 w425] -> w420
                        tunnel: w418 -> [_ w423]
                        tunnel: w415 -> [w421 w426]
                        frame False {
                        }
                        frame True {
                          # "Resetting at the end of every cycle"
                          # "Ramp Dn"
                          n163 = local write "Up/Down"(TRUE ("Up/Down")) -> ()
                          n164 = local read "Magnet"() -> (w422:bool)
                          n165 = local write "Target Field"(w423) -> ()
                          n166 = local write "Reset"(TRUE ("Reset")) -> ()
                          n167 = case shown="True" w422 {
                            tunnel: w426 -> [w428 w431]
                            tunnel: [w428 w430] -> w425
                            tunnel: w423 -> [_ w429]
                            frame False {
                            }
                            frame True {
                              n168 = call "Set_B.vi"("error in (no error)"=w431, "address string"="25", "Set Field (T)"=w429) -> ("error out"=w430:errorcluster)  [unwired: 8 in]
                            }
                          }
                        }
                      }
                      n169 = local write "Read?"(FALSE ("Read?")) -> ()
                    }
                  }
                }
                frame True {
                  n170 = local read "Setpoint Temperature (K)"() -> (w435:dbl)
                  n171 = local read "Min Temperature (K)"() -> (w434:dbl)
                  n172 = local read "Read?"() -> (w440:bool)
                  n173 = local read "Max temperature (K)"() -> (w433:dbl)
                  n174 = Equal?(x=w435, y=w434) -> (x = y?=w438:bool)
                  n175 = And(x=w438, y=w440) -> (x .and. y?=w439:bool)
                  n176 = case shown="True" w439 {
                    tunnel: [w446 w482] -> w436
                    tunnel: w433 -> [w454 w481]
                    tunnel: w434 -> [_ w480]
                    tunnel: w435 -> [_ w478]
                    tunnel: w437 -> [w447 w477]
                    frame True {
                      # "Ramp Up"
                      n177 = local read "First?"() -> (w457:bool)
                      n178 = case shown="True" w457 {
                        tunnel: [TRUE ("Save") FALSE ("Save")] -> w449
                        tunnel: [w469 w475] -> w452
                        frame False {
                          n179 = local read "Counter"() -> (w472:i8)
                          n180 = local write "Actual Polarization"(0.0 ("Actual Polarization")) -> ()
                          n181 = Increment(x=w472) -> (x+1=w469:i8)
                          n182 = local write "Counter"(w469) -> ()
                        }
                        frame True {
                          n183 = local read "Counter"() -> (w475:i8)
                          n184 = local write "First?"(FALSE ("First?")) -> ()
                        }
                      }
                      n185 = local write "Read?"(FALSE ("Read?")) -> ()
                      n186 = Number To Fractional String(number=w454, precision (6)=i16 3) -> (F-format string=w443:string)  [unwired: 2 in]
                      n187 = local read "Heater 2/1"() -> (w441:bool)
                      n188 = local read "Record ALL"() -> (w453:bool)
                      n189 = case shown="True" w453 {
                        tunnel: w452 -> [_ w468]
                        tunnel: [FALSE w467] -> w450
                        frame False {
                        }
                        frame True {
                          n190 = local read "Max Countl"() -> (w466:i32)
                          n191 = Greater?(x=w468, y=w466) -> (0:w467:bool)
                        }
                      }
                      n192 = local write "Reset"(w449) -> ()
                      n193 = Select(t="1,  " ("write buffer"), s=w441, f="2,  " ("write buffer")) -> (s? t:f=w442:string)
                      n194 = Concatenate Strings("SETP " ("write buffer"), w442, w443) -> (w448:string)
                      n195 = case shown="True" w450 {
                        tunnel: w448 -> [w462 _]
                        tunnel: w447 -> [w460 w463]
                        tunnel: [w459 w463] -> w446
                        frame False {
                          n196 = local read "Lake Shore"() -> (w461:refnum<visa-resource-name>)
                          n197 = VISA Write(VISA resource name=w461, write buffer=w462, error in (no error)=w460) -> (error out=w459:errorcluster)  [unwired: 2 out]
                        }
                        frame True {
                          n198 = local write "New"(TRUE ("New")) -> ()
                        }
                      }
                      "Up/Down 2" <- FALSE ("Up/Down")
                    }
                    frame False {
                      n199 = Equal?(x=w481, y=w478) -> (x = y?=w479:bool)
                      n200 = case shown="True" w479 {
                        tunnel: [w483 w494] -> w482
                        tunnel: w480 -> [_ w493]
                        tunnel: w477 -> [w483 w495]
                        frame False {
                        }
                        frame True {
                          w491 = TRUE ("Reset")
                          # "Ramp Dn"
                          n201 = local write "Up/Down 2"(w491) -> ()
                          n202 = Number To Fractional String(number=w493, precision (6)=i16 3) -> (F-format string=w487:string)  [unwired: 2 in]
                          n203 = local write "Reset"(w491) -> ()
                          n204 = local read "Lake Shore"() -> (w492:refnum<visa-resource-name>)
                          n205 = local read "Heater 2/1"() -> (w484:bool)
                          n206 = Select(t="1,  " ("write buffer"), s=w484, f="2,  " ("write buffer")) -> (s? t:f=w486:string)
                          n207 = Concatenate Strings("SETP " ("write buffer"), w486, w487) -> (w485:string)
                          n208 = VISA Write(VISA resource name=w492, write buffer=w485, error in (no error)=w495) -> (error out=w494:errorcluster)  [unwired: 2 out]
                        }
                      }
                      n209 = local write "Read?"(FALSE ("Read?")) -> ()
                    }
                  }
                }
              }
              n210 = local read "Magnet"() -> (w360:bool)
              n211 = case shown="True" w360 {
                tunnel: [Mode."StepDelta" ("Enum") Mode."Plot" ("Enum")] -> w362
                frame False {
                }
                frame True {
                }
              }
            }
            frame "StepDelta" {
              n212 = flat-sequence {
                tunnel: w498 -> [w513]
                tunnel: [w512] -> w497
                frame #0 {
                  # "Check if it is time to step Field"
                  n213 = local read "Sweep Rate (T/min)"() -> (w514:dbl)
                  n214 = local read "Time Lag"() -> (w510:dbl)
                  n215 = xnode "Sweep Delay"("SweepRate"=w514, "Resolution"=0.001 ("Voltage Step (V)")) -> ("Result"=w511:dbl)  [unwired: 2 in, 1 out]
                  n216 = Divide(x=w510, y=w511) -> (x/y=w508:dbl)
                  n217 = Multiply(x=0.001 ("y"), y=w508) -> (x*y=w507:dbl)
                  "deltaUaux" <- w507
                  n218 = stacked-sequence {
                    tunnel: w513 -> [_ w525]
                    tunnel: [_ w524] -> w512
                    tunnel: w507 -> [w519 _]
                    frame #0 {
                      n219 = local read "Hall Resistance (Ohm)"() -> (w522:dbl)
                      n220 = local read "Up/Down"() -> (w523:bool)
                      n221 = Add(x=w522, y=w519) -> (x+y=w521:dbl)
                      n222 = Subtract(x=w522, y=w519) -> (x-y=w520:dbl)
                      n223 = local read "Calibration Curve Data"() -> (w518:dbl[][])
                      n224 = Select(t=w520, s=w523, f=w521) -> (s? t:f=w516:dbl)
                      "Hall Resistance (Ohm)" <- w516
                      n225 = call "HallR_to_B.vi"("Measured R(Ohm)"=w516, "Calibration Curve Data"=w518) -> ("Interpolated B value"=w517:dbl)  [unwired: 9 in]
                      n226 = local write "Nominal Field (T)"(w517) -> ()
                    }
                    frame #1 {
                      n227 = local read "Hall Resistance (Ohm)"() -> (w530:dbl)
                      n228 = local read "Lock_in_Amplifier"() -> (w526:refnum<visa-resource-name>)
                      n229 = Format Into String(w530) -> (resulting string=w529:string)  [unwired: 3 in, 1 out]
                      n230 = Concatenate Strings("AUXV 1,", w529) -> (w527:string)
                      n231 = VISA Write(VISA resource name=w526, write buffer=w527, error in (no error)=w525) -> (error out=w524:errorcluster)  [unwired: 2 out]
                    }
                  }
                }
              }
            }
            frame "Plot" {
              # "dI"
              n232 = local read "Nominal Field (T)"() -> (w550:dbl)
              n233 = local read "Actual B Field (T)"() -> (w549:dbl)
              n234 = local read "P(uC/mm^2)"() -> (w552:dbl[])
              n235 = local read "B lag"() -> (w545:cluster{dbl[], dbl[]})
              n236 = local read "Actual Polarization"() -> (w551:dbl)
              n237 = Unbundle(w545) -> (w544:dbl[], w543:dbl[])
              n238 = Build Array (concatenate)(w543, w549) -> (w547:dbl[])
              n239 = Build Array (concatenate)(w544, w550) -> (w548:dbl[])
              n240 = local read "Actual Current (pA)"() -> (w553:dbl)
              n241 = local read "Time Lag"() -> (w565:dbl)
              n242 = Bundle(w548, w547) -> (→"B lag":cluster{dbl[], dbl[]})  [unwired: 1 in]
              n243 = Multiply(x=w553, y=w565) -> (x*y=w557:dbl)
              n244 = Divide(x=w557, y="Sample area (mm^2)") -> (x/y=w556:dbl)
              n245 = Add(x=w556, y=w551) -> (x+y=w555:dbl)
              "Actual Polarization" <- w555
              n246 = local read "Temp/Magnetic Field"() -> (w566:bool)
              n247 = Build Array (concatenate)(w552, w555) -> (→"P(uC/mm^2)":dbl[])
              n248 = case shown="False" w566 {
                tunnel: w563 -> [_ w626]
                tunnel: w560 -> [_ w608]
                tunnel: w555 -> [w573 w609]
                frame False {
                  # "Magnetic Field plotting"
                  n249 = local read "Up/Down"() -> (w578:bool)
                  n250 = case shown="True" w578 {
                    frame True {
                      # "Down"
                      n251 = local read "I(B) 3"() -> (w588:cluster{dbl[], dbl[]}[])
                      n252 = local read "I(B) 3"() -> (w592:cluster{dbl[], dbl[]}[])
                      n253 = Index Array(array=w588, index=1) -> (element=w586:cluster{dbl[], dbl[]})
                      n254 = Unbundle(w586) -> (w585:dbl[], w584:dbl[])
                      n255 = Index Array(array=w592, index=i8 0 ("t")) -> (element=w589:cluster{dbl[], dbl[]})
                      n256 = local read "Actual Current (pA)"() -> (w579:dbl)
                      n257 = local read "Actual B Field (T)"() -> (w581:dbl)
                      n258 = Build Array (concatenate)(w585, w581) -> (w583:dbl[])
                      n259 = Build Array (concatenate)(w584, w579) -> (w582:dbl[])
                      n260 = Bundle(w583, w582) -> (w580:cluster{dbl[], dbl[]})  [unwired: 1 in]
                      n261 = Build Array(w589, w580) -> (w590:cluster{dbl[], dbl[]}[])
                      n262 = local write "I(B) 3"(w590) -> ()
                    }
                    frame False {
                      # "Up"
                      n263 = local read "I(B) 3"() -> (w604:cluster{dbl[], dbl[]}[])
                      n264 = local read "I(B) 3"() -> (w606:cluster{dbl[], dbl[]}[])
                      n265 = Index Array(array=w604, index=0) -> (element=w602:cluster{dbl[], dbl[]})
                      n266 = Unbundle(w602) -> (w601:dbl[], w600:dbl[])
                      n267 = Index Array(array=w606, index=i8 1 ("t")) -> (element=w595:cluster{dbl[], dbl[]})
                      n268 = local read "Actual B Field (T)"() -> (w596:dbl)
                      n269 = Build Array (concatenate)(w601, w596) -> (w599:dbl[])
                      n270 = local read "Actual Current (pA)"() -> (w593:dbl)
                      n271 = Build Array (concatenate)(w600, w593) -> (w598:dbl[])
                      n272 = Bundle(w599, w598) -> (w597:cluster{dbl[], dbl[]})  [unwired: 1 in]
                      n273 = Build Array(w597, w595) -> (w594:cluster{dbl[], dbl[]}[])
                      n274 = local write "I(B) 3"(w594) -> ()
                    }
                  }
                  n275 = local read "Actual B Field (T)"() -> (w575:dbl)
                  n276 = local read "P(B)"() -> (w577:cluster{"yi":dbl[], dbl[]})
                  n277 = Unbundle(w577) -> ("yi"=w576:dbl[], w574:dbl[])
                  n278 = Build Array (concatenate)(w576, w575) -> (w572:dbl[])
                  n279 = Build Array (concatenate)(w574, w573) -> (w571:dbl[])
                  n280 = Bundle(w572, w571) -> (→"P(B)":cluster{dbl[], dbl[]})  [unwired: 1 in]
                }
                frame True {
                  # "Temperature plotting"
                  n281 = Quotient & Remainder(x=w626, y="Save Period") -> (x-y*floor(x/y)=w607:dbl)  [unwired: 1 out]
                  n282 = Greater?(x=w608, y=w607) -> (0:w624:bool)
                  n283 = local read "Actual Temperature (K)"() -> (w611:dbl)
                  n284 = local read "Actual Current (pA)"() -> (w617:dbl)
                  n285 = local read "P(T)"() -> (w613:cluster{"yi":dbl[], dbl[]})
                  n286 = local read "I(T)"() -> (w623:cluster{dbl[], dbl[]})
                  n287 = case shown="True" w624 {
                    frame False {
                    }
                    frame True {
                      n288 = local write "Reset"(TRUE) -> ()
                    }
                  }
                  n289 = Unbundle(w613) -> ("yi"=w614:dbl[], w610:dbl[])
                  n290 = Unbundle(w623) -> (w621:dbl[], w620:dbl[])
                  n291 = Build Array (concatenate)(w614, w611) -> (w615:dbl[])
                  n292 = Build Array (concatenate)(w610, w609) -> (w616:dbl[])
                  n293 = Build Array (concatenate)(w621, w611) -> (w619:dbl[])
                  n294 = Build Array (concatenate)(w620, w617) -> (w618:dbl[])
                  n295 = Bundle(w619, w618) -> (→"I(T)":cluster{dbl[], dbl[]})  [unwired: 1 in]
                  n296 = Bundle(w615, w616) -> (→"P(T)":cluster{dbl[], dbl[]})  [unwired: 1 in]
                }
              }
            }
            frame "Save" {
              n297 = local read "Reset"() -> (w628:bool)
              n298 = case shown="True" w628 {
                tunnel: w633 -> [w650 w652]
                tunnel: [w650 w655] -> w638
                tunnel: w632 -> [w649 w653]
                tunnel: [w649 w655] -> w637
                tunnel: w634 -> [w648 w654]
                tunnel: [w648 w655] -> w636
                tunnel: [w647 w655] -> w635
                tunnel: w631 -> [w647 w651]
                frame False {
                }
                frame True {
                  n299 = stacked-sequence {
                    tunnel: [_ _ w737] -> w655
                    tunnel: w654 -> [_ w726 _]
                    tunnel: w653 -> [w658 w724 _]
                    tunnel: w652 -> [w659 w725 _]
                    tunnel: w651 -> [w657 w722 _]
                    frame #0 {
                      n300 = local read "Temp/Magnetic Field"() -> (w656:bool)
                      n301 = case shown="False" w656 {
                        tunnel: w659 -> [w686 w713]
                        tunnel: w658 -> [w685 w712]
                        tunnel: w657 -> [w676 w703]
                        frame False {
                          n302 = local read "B array"() -> (w670:dbl[])
                          n303 = local read "Counter"() -> (w684:i8)
                          n304 = local read "Averaged I(B)"() -> (w661:dbl[][])
                          n305 = local read "Up/Down"() -> (w687:bool)
                          n306 = local read "Sample area (mm^2)"() -> (w666:dbl)
                          n307 = call "Average_IBP_curves_baseline.vi"("I in"=w685, "Averaged P(B) In"="Averaged P(B)", "Counter"=w684, "B0"="Threshold B (T)", "Averaged I(B) In"=w661, "t in"=w676, "B in"=w686, "Averaged dt in"="Averaged dt", "Up/Down"=w687, "Sample area(mm^2)"=w666, "B array"=w670) -> ("Averaged dt Out"=w673:dbl[][], "Averaged P(B) Out"=w662:dbl[][], "BaselineSubtracted I(B)"=w660:dbl[][])  [unwired: 1 in, 1 out]
                          "Averaged I(B)" <- w660
                          n308 = Index Array(array=w662, index (row)=0 ("disabled index (col)")) -> (element=w671:dbl[])  [unwired: 1 in]
                          n309 = Index Array(array=w662, index (row)=1 ("disabled index (col)")) -> (element=w672:dbl[])  [unwired: 1 in]
                          n310 = Index Array(array=w660, index (row)=0 ("disabled index (col)")) -> (element=w678:dbl[])  [unwired: 1 in]
                          n311 = Index Array(array=w660, index (row)=1 ("disabled index (col)")) -> (element=w677:dbl[])  [unwired: 1 in]
                          n312 = local write "Averaged dt"(w673) -> ()
                          n313 = Bundle("B array"=w670, "Averaged P(B) Out"=w671) -> (w669:T7)  [unwired: 1 in]
                          n314 = Bundle("B array"=w670, "Averaged P(B) Out"=w672) -> (w668:T7)  [unwired: 1 in]
                          n315 = local write "Averaged P(B)"(w662) -> ()
                          n316 = Bundle("B array"=w670, "BaselineSubtracted I(B)"=w678) -> (w683:T8)  [unwired: 1 in]
                          n317 = Bundle("B array"=w670, "BaselineSubtracted I(B)"=w677) -> (w682:T8)  [unwired: 1 in]
                          n318 = Build Array(w669, w668) -> (→"P(B) /Averaged/":T9)
                          n319 = Build Array(w683, w682) -> (→"I(B) /Averaged/":T10)
                        }
                        frame True {
                          n320 = local read "T array"() -> (w698:dbl[])
                          n321 = local read "Counter"() -> (w711:i8)
                          n322 = local read "Averaged I(T)"() -> (w690:dbl[][])
                          n323 = local read "Up/Down"() -> (w714:bool)
                          n324 = local read "Averaged dt"() -> (w689:dbl[][])
                          n325 = local read "Sample area (mm^2)"() -> (w694:dbl)
                          n326 = call "Average_ITP_curves.vi"("I in"=w712, "Averaged P(T) In"="Averaged P(T)", "Counter"=w711, "Averaged I(T) In"=w690, "t in"=w703, "T in"=w713, "Averaged dt in"=w689, "Up/Down"=w714, "Sample area(mm^2)"=w694, "T array"=w698) -> ("Averaged I(B) out"=w688:dbl[][], "Averaged dt Out"=w701:dbl[][], "Averaged P(T) Out"=w691:dbl[][])  [unwired: 3 in]
                          "Averaged I(T)" <- w688
                          n327 = Index Array(array=w691, index (row)=0 ("disabled index (col)")) -> (element=w699:dbl[])  [unwired: 1 in]
                          n328 = Index Array(array=w691, index (row)=1 ("disabled index (col)")) -> (element=w700:dbl[])  [unwired: 1 in]
                          n329 = Index Array(array=w688, index (row)=0 ("disabled index (col)")) -> (element=w705:dbl[])  [unwired: 1 in]
                          n330 = Index Array(array=w688, index (row)=1 ("disabled index (col)")) -> (element=w704:dbl[])  [unwired: 1 in]
                          n331 = local write "Averaged dt"(w701) -> ()
                          n332 = Bundle("T array"=w698, "Averaged P(T) Out"=w699) -> (w697:T11)  [unwired: 1 in]
                          n333 = Bundle("T array"=w698, "Averaged P(T) Out"=w700) -> (w696:T11)  [unwired: 1 in]
                          n334 = local write "Averaged P(T)"(w691) -> ()
                          n335 = Bundle("T array"=w698, "Averaged I(B) out"=w705) -> (w710:T12)  [unwired: 1 in]
                          n336 = Bundle("T array"=w698, "Averaged I(B) out"=w704) -> (w709:T12)  [unwired: 1 in]
                          n337 = Build Array(w697, w696) -> (→"P(T) /Averaged/":T13)
                          n338 = Build Array(w710, w709) -> (→"I(T) /Averaged/":T14)
                        }
                      }
                    }
                    frame #1 {
                      # "Save and Reset"
                      n339 = local read "Sweep"() -> (w715:bool)
                      n340 = local read "Measurement File"() -> (w717:path)
                      n341 = local read "P(uC/mm^2)"() -> (w723:dbl[])
                      n342 = Build Array(w726, w725, w724, w722, w723) -> (w716:dbl[][])
                      n343 = case shown="True" w715 {
                        tunnel: w716 -> [_ w733]
                        frame False {
                        }
                        frame True {
                          n344 = local read "Up/Down"() -> (w729:bool)
                          n345 = case shown="True" w729 {
                            tunnel: [w734 w735] -> w728
                            frame False {
                              n346 = local read "Measurement File_dn"() -> (w734:path)
                            }
                            frame True {
                              n347 = local read "Measurement File_up"() -> (w735:path)
                            }
                          }
                          n348 = call-poly <vilib>:"Write Delimited Spreadsheet.vi"("file path (dialog if empty)"=w728, "format (%.3f)"="%.5g", "2D data"=w733, "append to file? (F)"=TRUE ("transpose? (F)"), "transpose? (F)"=FALSE ("append to file? (F)")) -> ()  [unwired: 9 in, 2 out]
                        }
                      }
                      n349 = case shown="False" "Reset IB?" {
                        frame False {
                        }
                        frame True {
                          n350 = local read "Up/Down"() -> (w736:bool)
                          n351 = case shown="False" w736 {
                            frame False {
                              n352 = invoke on="I(B) 3" class="XYGraph (strict)" method="Reinit To Default"() -> ()  [unwired: 3 in, 3 out]
                              n353 = invoke on="I(T)" class="XYGraph (strict)" method="Reinit To Default"() -> ()  [unwired: 3 in, 3 out]
                            }
                            frame True {
                            }
                          }
                        }
                      }
                      n354 = call-poly <vilib>:"Write Delimited Spreadsheet.vi"("file path (dialog if empty)"=w717, "format (%.3f)"="%.5g", "2D data"=w716, "append to file? (F)"=TRUE, "transpose? (F)"=TRUE) -> ()  [unwired: 9 in, 2 out]
                      n355 = local write "Reset"(FALSE ("Save")) -> ()
                    }
                    frame #2 {
                      w737 = dbl[] []
                      n356 = local write "P(uC/mm^2)"(w737) -> ()
                    }
                  }
                }
              }
              n357 = local read "New"() -> (w630:bool)
              n358 = case shown="False" w630 {
                tunnel: [Mode."Return" ("Enum") Mode."New" ("Enum")] -> w642
                tunnel: [TRUE FALSE] -> w629
                frame False {
                }
                frame True {
                }
              }
            }
            frame "New" {
              n359 = local read "Temp/Magnetic Field"() -> (w738:bool)
              n360 = stacked-sequence {
                seq-local: [_ _ _ _ w877 _ _] -> [_ _ _ _ _ w906 _]
                seq-local: [_ _ w805 _ _ _ _] -> [_ _ _ w843 _ _ _]
                seq-local: [_ _ _ w844 _ _ _] -> [_ _ _ _ w876 _ _]
                tunnel: T6 {"Com Port"=1, "ISOBUS Address"=0, "GPIB Address"=25, "Communication"=enum."GPIB"} ("Address") -> [_ _ w804 w845 _ _ _]
                tunnel: w741 -> [_ _ w806 _ _ w907 _]
                tunnel: [_ _ _ _ _ w909 _] -> w740
                tunnel: w739 -> [_ w775 _ _ _ _ _]
                tunnel: w738 -> [_ _ w795 w842 w875 w905 _]
                frame #0 {
                  w767 = 1 ("index (row)")
                  w766 = 0 ("index (row)")
                  # "Save averages"
                  n361 = local read "Measurement File_average"() -> (w754:path)
                  n362 = local read "Averaged P(B)"() -> (w765:dbl[][])
                  n363 = local read "Averaged dt"() -> (w763:dbl[][])
                  n364 = local read "I(B) /Averaged/"() -> (w755:cluster{"B array":dbl[], dbl[]}[])
                  n365 = Index Array(array=w763, index (row)=w766) -> (element=w764:dbl[])  [unwired: 1 in]
                  n366 = Index Array(array=w763, index (row)=w767) -> (element=w771:dbl[])  [unwired: 1 in]
                  n367 = Index Array(array=w755, index=1) -> (element=w759:cluster{"B array":dbl[], dbl[]})
                  n368 = Index Array(array=w755, index=0) -> (element=w758:cluster{"B array":dbl[], dbl[]})
                  n369 = Unbundle(w759) -> ("B array"=w769:dbl[], w770:dbl[])
                  n370 = Unbundle(w758) -> ("B array"=w760:dbl[], w761:dbl[])
                  n371 = Index Array(array=w765, index (row)=w766) -> (element=w768:dbl[])  [unwired: 1 in]
                  n372 = Index Array(array=w765, index (row)=w767) -> (element=w772:dbl[])  [unwired: 1 in]
                  n373 = Build Array(w760, w761, w764, w768, w769, w770, w771, w772) -> (w762:dbl[][])
                  n374 = call-poly <vilib>:"Write Delimited Spreadsheet.vi"("file path (dialog if empty)"=w754, "format (%.3f)"="%.5g", "2D data"=w762, "append to file? (F)"=TRUE ("transpose? (F)"), "transpose? (F)"=TRUE ("append to file? (F)")) -> ()  [unwired: 9 in, 2 out]
                }
                frame #1 {
                  w781 = dbl[] []
                  w789 = dbl[] []
                  # "Reset Flags"
                  n375 = Get Date/Time In Seconds() -> (seconds since 1Jan1904=w790:timestamp)
                  n376 = local write "Up/Down"(TRUE ("Up/Down")) -> ()
                  n377 = local write "First?"(TRUE ("First?")) -> ()
                  n378 = local write "New"(FALSE ("New")) -> ()
                  n379 = local write "P(uC/mm^2)"(w789) -> ()
                  n380 = local write "Start time"(w790) -> ()
                  n381 = local write "Actual Polarization"(0.0 ("Actual Polarization")) -> ()
                  n382 = local write "Offset array"(w789) -> ()
                  n383 = local write "Up/Down"(TRUE ("Up/Down")) -> ()
                  n384 = local write "Reset"(FALSE ("Reset")) -> ()
                  n385 = local write "Offset?"("Reoffset?") -> ()
                  n386 = local read "B array"() -> (w783:dbl[])
                  n387 = local write "Counter"(i8 0 ("Counter")) -> ()
                  n388 = invoke on="P(B)" class="XYGraph (strict)" method="Reinit To Default"() -> ()  [unwired: 3 in, 3 out]
                  n389 = invoke on="I(B) 3" class="XYGraph (strict)" method="Reinit To Default"() -> ()  [unwired: 3 in, 3 out]
                  n390 = Multiply(x=w783, y=0.0) -> (x*y=w784:dbl[])
                  n391 = Build Array(w781, w781) -> (w788:dbl[][])
                  n392 = Bundle("B array"=w783, w784) -> (w785:cluster{"B array":dbl[], dbl[]})  [unwired: 1 in]
                  n393 = local write "Averaged I(B)"(w788) -> ()
                  n394 = Build Array(w785, w785) -> (w786:cluster{"B array":dbl[], dbl[]}[])
                  n395 = local write "I(B) /Averaged/"(w786) -> ()
                  n396 = local write "Measuring"(FALSE ("Measuring")) -> ()
                  n397 = Flush Queue(queue=w775) -> (remaining elements=→"remaining elements 2":T1)  [unwired: 1 in, 2 out]
                }
                frame #2 {
                  # "Step"
                  n398 = local read "T Sweep Rate Array"() -> (w800:dbl[])
                  n399 = local read "Sweep Rate Array"() -> (w799:dbl[])
                  n400 = local read "Temperature Array"() -> (w796:dbl[])
                  n401 = local read "Magnetic Field array (T)"() -> (w797:dbl[])
                  n402 = local read "Heater 2/1"() -> (w793:bool)
                  n403 = local read "j"() -> (w810:i32)
                  n404 = Increment(x=w810) -> (x+1=w807:i32)
                  n405 = Select(t=w800, s=w795, f=w799) -> (s? t:f=w798:dbl[])
                  n406 = Array Size(array=w798) -> (size(s)=w809:i32)
                  n407 = Less?(x=w807, y=w809) -> (x < y?=w808:bool)
                  "Step Rate" <- w808
                  n408 = Select(t="1,0  " ("write buffer"), s=w793, f="2,0  " ("write buffer")) -> (s? t:f=w801:string)
                  n409 = Select(t=w797, s=w795, f=w796) -> (s? t:f=w794:dbl[])
                  n410 = case shown="False" w808 {
                    tunnel: w807 -> [_ w841]
                    tunnel: w806 -> [w815 w840]
                    tunnel: [w814 w840] -> w805
                    tunnel: w804 -> [w813 _]
                    tunnel: w801 -> [w812 _]
                    tunnel: w794 -> [w811 _]
                    frame False {
                      # "Step Temp?"
                      n411 = local read "i"() -> (w819:i32)
                      n412 = Increment(x=w819) -> (x+1=w817:i32)
                      n413 = local write "j"(0 ("f")) -> ()
                      n414 = Array Size(array=w811) -> (size(s)=w818:i32)
                      n415 = Less?(x=w817, y=w818) -> (x < y?=w816:bool)
                      "Step Temp" <- w816
                      n416 = case shown="False" w816 {
                        tunnel: w817 -> [_ w839]
                        tunnel: w815 -> [w825 w838]
                        tunnel: [w824 w838] -> w814
                        tunnel: w813 -> [w823 _]
                        tunnel: w812 -> [w821 _]
                        frame False {
                          # "Heater OFF"
                          # "Finished"
                          n417 = local write "i"(0 ("i")) -> ()
                          n418 = stacked-sequence {
                            tunnel: w825 -> [w832 _ _]
                            tunnel: [w831 _ _] -> w824
                            tunnel: w823 -> [_ w835 w836]
                            tunnel: w821 -> [w829 _ _]
                            frame #0 {
                              n419 = Concatenate Strings("RANGE," ("write buffer"), w829) -> (w828:string)
                              n420 = local read "Lake Shore"() -> (w833:refnum<visa-resource-name>)
                              n421 = VISA Write(VISA resource name=w833, write buffer=w828, error in (no error)=w832) -> (error out=w831:errorcluster)  [unwired: 2 out]
                            }
                            frame #1 {
                              n422 = call "ips_switchHeaterOff.vi"("Instrument address"=w835, "Rate"=2.0) -> ()  [unwired: 1 out]
                            }
                            frame #2 {
                              n423 = call "GPIB - BusCommand.vi"("Command"="H0", "Address"=w836) -> ()  [unwired: 2 out]
                            }
                          }
                          n424 = local write "Record ALL"(FALSE ("Record ALL")) -> ()
                          "Finished" <- TRUE
                        }
                        frame True {
                          n425 = local write "i"(w839) -> ()
                        }
                      }
                    }
                    frame True {
                      n426 = local write "j"(w841) -> ()
                    }
                  }
                }
                frame #3 {
                  # "Set rates"
                  n427 = case shown="True" w842 {
                    tunnel: w845 -> [w853 _]
                    tunnel: w843 -> [w846 w861]
                    tunnel: [w846 w860] -> w844
                    frame False {
                      n428 = local read "Sweep Rate Array"() -> (w852:dbl[])
                      n429 = local read "j"() -> (w851:i32)
                      n430 = local read "j"() -> (w849:i32)
                      n431 = Index Array(array=w852, index=w851) -> (element=w850:dbl)
                      n432 = Number To Fractional String(number=w850, precision (6)=i16 3) -> (F-format string=w856:string)  [unwired: 2 in]
                      n433 = Index Array(array="Max count array", index=w849) -> (element=w847:i32)
                      n434 = local write "Max Countl"(w847) -> ()
                      n435 = Concatenate Strings("T" ("format string"), w856) -> (w857:string)
                      n436 = call "GPIB - BusCommand.vi"("Command"=w857, "Address"=w853) -> ()  [unwired: 2 out]
                      n437 = local write "Sweep Rate (T/min)"(w850) -> ()
                    }
                    frame True {
                      n438 = local read "T Sweep Rate Array"() -> (w870:dbl[])
                      n439 = local read "Max count array"() -> (w868:i32[])
                      n440 = local read "j"() -> (w873:i32)
                      n441 = local read "j"() -> (w872:i32)
                      n442 = Index Array(array=w870, index=w873) -> (element=w869:dbl)
                      n443 = Number To Fractional String(number=w869, precision (6)=i16 1) -> (F-format string=w863:string)  [unwired: 2 in]
                      n444 = Index Array(array=w868, index=w872) -> (element=w871:i32)
                      n445 = local read "Heater 2/1"() -> (w858:bool)
                      n446 = local write "Max Countl"(w871) -> ()
                      n447 = local write "Temp Ramping Rate (K/min)"(w869) -> ()
                      n448 = Select(t="1,1,  " ("write buffer"), s=w858, f="2,1,  " ("write buffer")) -> (s? t:f=w864:string)
                      n449 = local read "Lake Shore"() -> (w859:refnum<visa-resource-name>)
                      n450 = Concatenate Strings("RAMP " ("string"), w864, w863) -> (w862:string)
                      n451 = VISA Write(VISA resource name=w859, write buffer=w862, error in (no error)=w861) -> (error out=w860:errorcluster)  [unwired: 2 out]
                    }
                  }
                }
                frame #4 {
                  # "Set temperature"
                  n452 = case shown="False" w875 {
                    tunnel: [w892 w899] -> w877
                    tunnel: w876 -> [w885 w900]
                    frame False {
                      n453 = local read "Temperature Array"() -> (w896:dbl[])
                      n454 = local read "Heater Range Array"() -> (w879:i8[])
                      n455 = local read "i"() -> (w884:i32)
                      n456 = Index Array(array=w896, index=w884) -> (element=w895:dbl)
                      n457 = local read "Heater 2/1"() -> (w878:bool)
                      n458 = local read "Lake Shore"() -> (w897:refnum<visa-resource-name>)
                      n459 = Index Array(array=w879, index=w884) -> (element=w880:i8)
                      n460 = Number To Fractional String(number=w895, precision (6)=i16 3) -> (F-format string=w888:string)  [unwired: 2 in]
                      n461 = Select(t="1,  " ("write buffer"), s=w878, f="2,  " ("write buffer")) -> (s? t:f=w886:string)
                      n462 = Concatenate Strings("SETP " ("write buffer"), w886, w888) -> (w887:string)
                      n463 = VISA Write(VISA resource name=w897, write buffer=w887, error in (no error)=w885) -> (VISA resource name out=w894:refnum<visa-resource-name>, error out=w893:errorcluster)  [unwired: 1 out]
                      n464 = Number To Decimal String(number=w880) -> (decimal integer string=w883:string)  [unwired: 1 in]
                      n465 = Concatenate Strings("RANGE," ("write buffer"), w886, w883) -> (w882:string)
                      n466 = VISA Write(VISA resource name=w894, write buffer=w882, error in (no error)=w893) -> (error out=w892:errorcluster)  [unwired: 2 out]
                    }
                    frame True {
                      n467 = local read "Magnetic Field array (T)"() -> (w903:dbl[])
                      n468 = local read "i"() -> (w904:i32)
                      n469 = Index Array(array=w903, index=w904) -> (element=w902:dbl)
                      n470 = call "Set_B.vi"("error in (no error)"=w900, "address string"="25", "Set Field (T)"=w902) -> ("error out"=w899:errorcluster)  [unwired: 8 in]
                    }
                  }
                }
                frame #5 {
                  n471 = local read "Finished"() -> (w908:bool)
                  n472 = case shown="False" w908 {
                    tunnel: [w938 w989] -> w909
                    tunnel: w907 -> [_ _]
                    tunnel: w906 -> [w935 w989]
                    tunnel: w905 -> [w913 _]
                    frame False {
                      w933 = "_" ("string")
                      # "Wait, create Files"
                      n473 = local read "Temperature Array"() -> (w924:dbl[])
                      n474 = local read "T Sweep Rate Array"() -> (w922:dbl[])
                      n475 = local read "Magnetic Field array (T)"() -> (w912:dbl[])
                      n476 = local read "Sweep Rate Array"() -> (w920:dbl[])
                      n477 = Select(t=w922, s=w913, f=w920) -> (s? t:f=w921:dbl[])
                      n478 = local read "i"() -> (w961:i32)
                      n479 = local read "j"() -> (w959:i32)
                      n480 = Multiply(x=w912, y=1000) -> (x*y=w910:dbl[])
                      n481 = Select(t=w910, s=w913, f=w924) -> (s? t:f=w923:dbl[])
                      n482 = Index Array(array=w923, index=w961) -> (element=w960:dbl)
                      n483 = Index Array(array=w921, index=w959) -> (element=w930:dbl)
                      n484 = Round Toward -Infinity(1:w930) -> (0:w931:dbl)
                      n485 = Number To Fractional String(use system decimal point (T)=TRUE, number=w960, precision (6)=i16 1) -> (F-format string=w925:string)  [unwired: 1 in]
                      n486 = Subtract(x=w930, y=w931) -> (x-y=w932:dbl)
                      n487 = Equal To 0?(x=w932) -> (x = 0?=w929:bool)
                      n488 = Select(t="mT", s=w913, f="K" ("string")) -> (s? t:f=w917:string)
                      n489 = Select(t=i16 0 ("precision (6)"), s=w929, f=i16 2 ("precision (6)")) -> (s? t:f=w926:i16)
                      n490 = Number To Fractional String(use system decimal point (T)=TRUE, number=w930, precision (6)=w926) -> (F-format string=w934:string)  [unwired: 1 in]
                      n491 = local read "Step Temp"() -> (w939:bool)
                      n492 = Select(t="Kpm" ("string"), s=w913, f="Tpm" ("string")) -> (s? t:f=w914:string)
                      n493 = Concatenate Strings("Directory", "\\" ("string"), "FileName", w933, w925, w917, w933, w934, w914) -> (w955:string)
                      n494 = local write "Step Rate"(FALSE ("Step Rate")) -> ()
                      n495 = Search and Replace String(replace all?=TRUE ("replace all? (F)"), input string=w955, search string=".", replace string="p" ("substring (\"\")"), error in=w935) -> (result string=w950:string, error out=w945:errorcluster)  [unwired: 3 in, 2 out]
                      n496 = Concatenate Strings(w950, ".txt" ("string")) -> (w949:string)
                      n497 = case shown="True" w939 {
                        tunnel: w925 -> [_ w964]
                        tunnel: w913 -> [_ w963]
                        frame False {
                        }
                        frame True {
                          n498 = stacked-sequence {
                            tunnel: w964 -> [_ w972 _]
                            tunnel: w963 -> [_ w971 w987]
                            frame #0 {
                              n499 = Get Date/Time In Seconds() -> (seconds since 1Jan1904=w965:timestamp)
                              n500 = while {
                                tunnel: w965 -> [w969]
                                stop <- w966 stop-if-true
                                n501 = Get Date/Time In Seconds() -> (seconds since 1Jan1904=w970:timestamp)
                                n502 = Subtract(x=w970, y=w969) -> (x-y=w968:dbl)
                                "Wait (s)" <- w968
                                n503 = Greater Or Equal?(x=w968, y="secs to wait") -> (x >= y?=w966:bool)
                              }
                            }
                            frame #1 {
                              n504 = case shown="False" w971 {
                                tunnel: w972 -> [w981 _]
                                frame False {
                                n505 = local read "Directory"() -> (w977:string)
                                n506 = local read "Max Field"() -> (w975:dbl)
                                n507 = Concatenate Strings(w977, "\\" ("string"), w981, "K_calib" ("string"), ".txt" ("string")) -> (w982:string)
                                n508 = local read "Start Field"() -> (w974:dbl)
                                n509 = String To Path(string=w982) -> (path=w979:path)
                                n510 = call "Calibration_Hall_full.vi"("Reset Field"=w974, "Min Field"=w974, "Max Field"=w975) -> ("Calibration Curve"=w986:cluster{dbl[], "Best Linear Fit":dbl[]}[], "Calibration Curve Data"=w983:dbl[][])  [unwired: 7 in]
                                n511 = Transpose 2D Array(2D array=w983) -> (transposed array=w984:dbl[][])
                                n512 = local write "Calibration Curve Data"(w983) -> ()
                                n513 = call-poly <vilib>:"Write Delimited Spreadsheet.vi"("file path (dialog if empty)"=w979, "format (%.3f)"="%.8f", "2D data"=w984) -> ()  [unwired: 11 in, 2 out]
                                n514 = local write "Calibration Curve"(w986) -> ()
                                }
                                frame True {
                                }
                              }
                              n515 = local write "Step Temp"(FALSE ("Step Temp")) -> ()
                            }
                            frame #2 {
                              n516 = case shown="False" w987 {
                                frame False {
                                n517 = Wait (ms)(milliseconds to wait=u32 20000) -> ()  [unwired: 1 out]
                                }
                                frame True {
                                }
                              }
                            }
                          }
                        }
                      }
                      n518 = String To Path(string=w949) -> (path=w948:path)
                      n519 = Open/Create/Replace File(file path (use dialog)=w948, error in=w945, operation (0:open)=T5."open or create") -> (refnum out=w937:refnum<file>, error out=w938:errorcluster)  [unwired: 3 in, 1 out]
                      n520 = local write "refnum out"(w937) -> ()
                      n521 = Refnum to Path(1:w937) -> (0:w940:path)
                      n522 = call "Create_sweep_files.vi"("Measurement File"=w940) -> ("Path 3"=w943:path, "Path 2"=w942:path, "Path"=w941:path)  [unwired: 8 in]
                      n523 = local write "Measurement File_average"(w941) -> ()
                      n524 = local write "Measurement File"(w940) -> ()
                      n525 = local write "Measurement File_dn"(w943) -> ()
                      n526 = local write "Measurement File_up"(w942) -> ()
                    }
                    frame True {
                    }
                  }
                }
                frame #6 {
                  n527 = local read "Finished"() -> (w990:bool)
                  n528 = case shown="False" w990 {
                    frame False {
                      n529 = local write "Measuring"(TRUE ("Measuring")) -> ()
                    }
                    frame True {
                      n530 = local write "Measure /Pause"(FALSE ("Measure /Pause")) -> ()
                    }
                  }
                }
              }
            }
            frame "Return" {
            }
          }
        }
      }
      frame Error {
        # "Return true for any case which should stop the loop."
      }
    }
  }
  "error out" <- w7
  n531 = VISA Read(VISA resource name=w26, byte count=u32 100, error in (no error)=w28) -> (VISA resource name out=w25:refnum<visa-resource-name>, read buffer=w24:string, error out=w27:errorcluster)  [unwired: 1 out]
  n532 = VISA Open(error in (no error)=w27, VISA resource name="Magnetic Field") -> (VISA resource name=w117:refnum<visa-resource-name>, error out=w100:errorcluster)  [unwired: 3 in]
  n533 = VISA Open(error in (no error)=w100, VISA resource name="Lake Shore") -> (VISA resource name=w95:refnum<visa-resource-name>, error out=w67:errorcluster)  [unwired: 3 in]
  n534 = VISA Write(VISA resource name="Lake Shore", write buffer=w13, error in (no error)=w67) -> (VISA resource name out=w64:refnum<visa-resource-name>, error out=w63:errorcluster)  [unwired: 1 out]
  n535 = VISA Read(VISA resource name=w64, byte count=w70, error in (no error)=w63) -> (VISA resource name out=w61:refnum<visa-resource-name>, read buffer=w74:string, error out=w62:errorcluster)  [unwired: 1 out]
  n536 = VISA Write(VISA resource name=w61, write buffer=w11, error in (no error)=w62) -> (VISA resource name out=w60:refnum<visa-resource-name>, error out=w59:errorcluster)  [unwired: 1 out]
  n537 = VISA Read(VISA resource name=w60, byte count=w70, error in (no error)=w59) -> (VISA resource name out=w57:refnum<visa-resource-name>, read buffer=w73:string, error out=w58:errorcluster)  [unwired: 1 out]
  n538 = VISA Write(VISA resource name=w57, write buffer=w8, error in (no error)=w58) -> (VISA resource name out=w55:refnum<visa-resource-name>, error out=w56:errorcluster)  [unwired: 1 out]
  n539 = Fract/Exp String To Number(string=w74) -> (number=w72:dbl)  [unwired: 3 in, 1 out]
  n540 = VISA Read(VISA resource name=w55, byte count=w70, error in (no error)=w56) -> (read buffer=w69:string, error out=w66:errorcluster)  [unwired: 2 out]
  n541 = Fract/Exp String To Number(string=w73) -> (number=w71:dbl)  [unwired: 3 in, 1 out]
  n542 = Fract/Exp String To Number(string=w69) -> (number=w65:dbl)  [unwired: 3 in, 1 out]
  n543 = local write "Actual Temperature (K)"(w72) -> ()
  n544 = local write "Setpoint Temperature (K)"(w71) -> ()
  n545 = local write "Heater Range"(w65) -> ()
  n546 = case shown="True" w77 {
    frame False {
    }
    frame True {
      n547 = invoke on="P(T)" class="XYGraph (strict)" method="Reinit To Default"() -> ()  [unwired: 3 in, 3 out]
      n548 = invoke on="I(T)" class="XYGraph (strict)" method="Reinit To Default"() -> ()  [unwired: 3 in, 3 out]
    }
  }
  n549 = Decimal String To Number(string=w24) -> (number=w23:i32)  [unwired: 2 in, 1 out]
  n550 = local write "Keithley (IV conv) averaging"(w23) -> ()
  n551 = while {
    shift-right: [w1021] -> w115
    shift-left: w97 -> [w1022]
    shift-right: [w1023] -> w120
    shift-left: w121 -> [w1024]
    tunnel: w25 -> [w1020]
    tunnel: w117 -> [w1019]
    tunnel: w66 -> [_]
    tunnel: [w1013] -> _
    tunnel: w105 -> [w1012]
    tunnel: w95 -> [w1011]
    tunnel: w33 -> [w1010]
    stop <- "stop" stop-if-true
    n552 = event shown="[0] Timeout" {
      selector: _ -> [_ _ _ _ _ _ _ _ _ _ _ _ _ _ _ _]
      dyn-events: _ -> [_ _ _ _ _ _ _ _ _ _ _ _ _ _ _ _]
      timeout: 10 -> [_ _ _ _ _ _ _ _ _ _ _ _ _ _ _ _]
      tunnel: w1024 -> [w1034 w1080 w1098 w1108 w1122 w1178 w1182 w1186 w1224 w1240 w1257 w1287 w1304 w1334 w1349 w1358]
      tunnel: [w1033 w1080 w1098 w1108 w1122 w1178 w1182 w1186 w1224 w1240 w1257 w1287 w1304 w1334 w1349 w1358] -> w1023
      tunnel: w1022 -> [w1032 w1089 w1097 w1107 w1120 w1177 w1184 w1188 w1225 w1239 w1256 w1288 w1306 w1338 w1353 w1360]
      tunnel: [w1031 w1081 w1097 w1107 w1119 w1179 w1184 w1187 _ w1239 w1256 w1288 w1305 w1337 w1352 w1359] -> w1021
      tunnel: w1020 -> [w1030 w1090 _ _ _ _ _ _ _ _ _ _ _ _ _ _]
      tunnel: w1019 -> [w1029 _ _ _ _ _ _ _ _ _ _ _ _ _ _ _]
      tunnel: [w1027 w1079 w1096 w1106 w1121 w1180 w1183 w1185 w1223 w1238 w1255 w1286 w1303 w1335 w1350 _] -> w1013
      tunnel: w1012 -> [w1027 w1079 w1096 w1109 w1121 w1180 w1183 w1185 w1223 w1238 w1255 w1286 w1303 w1335 w1350 _]
      tunnel: w1011 -> [_ _ _ _ _ _ _ _ _ _ _ _ w1307 w1336 w1354 w1357]
      tunnel: [_ _ _ _ _ _ _ _ w1225 _ _ _ _ _ _ _] -> _
      tunnel: w1010 -> [w1026 _ _ _ _ _ _ _ _ _ _ _ _ _ _ _]
      event Timeout {
        n553 = event-data() -> ()  [unwired: 1 in, 3 out]
        n554 = case shown="True" "Measuring" {
          tunnel: w1034 -> [w1036 w1059]
          tunnel: [w1036 w1058] -> w1033
          tunnel: w1032 -> [w1035 w1037]
          tunnel: [w1035 w1057] -> w1031
          tunnel: w1030 -> [_ w1050]
          tunnel: w1029 -> [_ w1049]
          tunnel: w1026 -> [_ w1040]
          frame False {
          }
          frame True {
            w1048 = ":FETCh? " ("data")
            w1051 = u32 1000 ("byte count")
            # "Generate the data here."
            n555 = case shown="No Error" w1037 {
              selector: w1037 -> [w1071 w1072]
              tunnel: [w1071 w1072] -> w1045
              tunnel: [w1070 _] -> w1044
              frame No Error {
                n556 = Get Date/Time In Seconds() -> (seconds since 1Jan1904=w1070:timestamp)
              }
              frame Error {
              }
            }
            n557 = VISA Write(VISA resource name=w1050, write buffer=w1048, error in (no error)=w1045) -> (VISA resource name out=w1056:refnum<visa-resource-name>, error out=w1054:errorcluster)  [unwired: 1 out]
            n558 = VISA Write(VISA resource name=w1049, write buffer=w1048, error in (no error)=w1054) -> (VISA resource name out=w1055:refnum<visa-resource-name>, error out=w1053:errorcluster)  [unwired: 1 out]
            n559 = VISA Read(VISA resource name=w1056, byte count=w1051, error in (no error)=w1053) -> (read buffer=w1046:string, error out=w1052:errorcluster)  [unwired: 2 out]
            n560 = VISA Read(VISA resource name=w1055, byte count=w1051, error in (no error)=w1052) -> (read buffer=w1047:string, error out=w1042:errorcluster)  [unwired: 2 out]
            n561 = case shown="False" "DaQ" {
              tunnel: w1042 -> [w1061 w1067]
              tunnel: [w1061 w1066] -> w1041
              tunnel: w1040 -> [_ w1065]
              tunnel: [0.0 ("Output") w1063] -> w1038
              frame False {
              }
              frame True {
                n562 = local read "Number of Samples"() -> (w1069:i32)
                n563 = call-poly <vilib>:"DAQmx Read.vi"("task/channels in"=w1065, "number of samples per channel"=w1069, "error in"=w1067) -> ("data"=w1068:dbl[], "error out"=w1066:errorcluster)  [unwired: 10 in, 1 out]
                n564 = call-poly <vilib>:"Mean.vi"("X"=w1068) -> ("mean"=w1064:dbl)  [unwired: 1 out]
                "Actual mean" <- w1064
                n565 = call "N Point Running Average.vi"("n"="Moving average", "Input"=w1064) -> ("Output"=w1063:dbl)
              }
            }
            n566 = Bundle("seconds since 1Jan1904"=w1044, "read buffer"=w1046, "read buffer"=w1047, "Output"=w1038) -> (w1043:T4)  [unwired: 1 in]
            n567 = Enqueue Element(queue=w1059, element=w1043, error in (no error)=w1041) -> (queue out=w1058:refnum<queue>, error out=w1057:errorcluster)  [unwired: 1 in, 1 out]
          }
        }
      }
      event "Keithley (IV conv) averaging": Value Change {
        n568 = event-data() -> ()  [unwired: 1 in, 6 out]
        n569 = Number To Decimal String(number="Keithley (IV conv) averaging") -> (decimal integer string=w1087:string)  [unwired: 1 in]
        n570 = Concatenate Strings("VOLTage:DC:AVERage:COUNt " ("write buffer"), w1087) -> (w1086:string)
        n571 = VISA Write(VISA resource name=w1090, write buffer=w1086, error in (no error)=w1089) -> (VISA resource name out=w1085:refnum<visa-resource-name>, error out=w1083:errorcluster)  [unwired: 1 out]
        n572 = VISA Write(VISA resource name=w1085, write buffer="VOLTage:DC:AVERage:COUNt?", error in (no error)=w1083) -> (VISA resource name out=w1078:refnum<visa-resource-name>, error out=w1082:errorcluster)  [unwired: 1 out]
        n573 = VISA Read(VISA resource name=w1078, byte count=u32 100, error in (no error)=w1082) -> (read buffer=w1076:string, error out=w1081:errorcluster)  [unwired: 2 out]
        n574 = Decimal String To Number(string=w1076) -> (number=w1075:i32)  [unwired: 2 in, 1 out]
        n575 = Equal?(x="Keithley (IV conv) averaging", y=w1075) -> (x = y?=→"Confirm":bool)
      }
      event "Max Field (T)": Value Change {
        n576 = event-data() -> ()  [unwired: 1 in, 6 out]
        n577 = Divide(x="Max Field (T)", y="dB (T)") -> (x/y=w1093:dbl)
        n578 = for {
          N: w1093 -> [_]
          tunnel: "dB (T)" -> [w1103]
          tunnel: [w1100] -> w1092 mode=indexing
          tunnel: "Min Field (T)" -> [w1101]
          tunnel: [0.0] -> _ mode=indexing
          i -> [w1104]
          n579 = Multiply(x=w1104, y=w1103) -> (x*y=w1102:dbl)
          n580 = Add(x=w1102, y=w1101) -> (x+y=w1100:dbl)
        }
        "B array" <- w1092
      }
      event "Sweep Rate (T/min)": Value Change {
        n581 = event-data() -> ("NewVal"=w1110:dbl)  [unwired: 1 in, 5 out]
        n582 = local read "Magnet"() -> (w1105:bool)
        n583 = case shown="False" w1105 {
          tunnel: w1110 -> [_ w1117]
          tunnel: w1109 -> [w1111 w1113]
          tunnel: [w1111 w1112] -> w1106
          frame False {
          }
          frame True {
            n584 = Number To Fractional String(number=w1117, precision (6)=i16 3) -> (F-format string=w1115:string)  [unwired: 2 in]
            n585 = Concatenate Strings("T" ("format string"), w1115) -> (w1114:string)
            n586 = call "GPIB - BusCommand.vi"("Command"=w1114, "Address"=w1113) -> ("Address(thru)"=w1112:T6)  [unwired: 1 out]
          }
        }
      }
      event "Field To Zero": Value Change {
        n587 = event-data() -> ()  [unwired: 1 in, 6 out]
        n588 = Two Button Dialog(message="Do you want to switch off the field?", 1:"No" ("F button name (\"Cancel\")"), 2:"Yes" ("T button name (\"OK\")")) -> (T button?=w1126:bool)
        n589 = case shown="True" w1126 {
          tunnel: w1121 -> [_ w1131]
          tunnel: w1120 -> [w1127 w1129]
          tunnel: [w1127 w1128] -> w1119
          frame False {
          }
          frame True {
            n590 = local read "Magnet"() -> (w1130:bool)
            n591 = case shown="False" w1130 {
              tunnel: w1131 -> [_ w1170]
              tunnel: w1129 -> [w1134 w1167]
              tunnel: [w1133 w1167] -> w1128
              frame False {
                n592 = local read "Lock_in_Amplifier"() -> (w1132:refnum<visa-resource-name>)
                n593 = stacked-sequence {
                  seq-local: [w1137 _] -> [_ w1150]
                  seq-local: [w1135 _] -> [_ w1147]
                  tunnel: w1134 -> [w1139 _]
                  tunnel: [_ w1151] -> w1133
                  tunnel: w1132 -> [w1136 w1148]
                  frame #0 {
                    n594 = VISA Write(VISA resource name=w1136, write buffer="AUXV?1", error in (no error)=w1139) -> (VISA resource name out=w1143:refnum<visa-resource-name>, error out=w1138:errorcluster)  [unwired: 1 out]
                    n595 = VISA Read(VISA resource name=w1143, byte count=u32 1000, error in (no error)=w1138) -> (read buffer=w1140:string, error out=w1137:errorcluster)  [unwired: 2 out]
                    n596 = Fract/Exp String To Number(string=w1140) -> (number=w1135:dbl)  [unwired: 3 in, 1 out]
                  }
                  frame #1 {
                    w1154 = 0.001 ("Voltage Step (V)")
                    n597 = local read "Sweep Rate (T/min)"() -> (w1153:dbl)
                    n598 = xnode "Sweep Delay"("SweepRate"=w1153, "Resolution"=w1154) -> ("Result"=w1152:dbl)  [unwired: 2 in, 1 out]
                    n599 = call "Universal_Ramping.vi"("milliseconds to wait"=w1152, "Initial Voltage (V)"=w1147, "error in (no error)"=w1150, "Voltage Step (V)"=w1154, "Final Voltage (V)"=0.0, "VISA resource name"=w1148) -> ("error out"=w1151:errorcluster, "Actual Voltage (V)"=w1144:dbl)  [unwired: 3 in, 1 out]
                    n600 = local read "Calibration Curve Data"() -> (w1146:dbl[][])
                    n601 = local write "Hall Resistance (Ohm)"(w1144) -> ()
                    n602 = call "HallR_to_B.vi"("Measured R(Ohm)"=w1144, "Calibration Curve Data"=w1146) -> ("Interpolated B value"=w1145:dbl)  [unwired: 9 in]
                    n603 = local write "Actual B Field (T)"(w1145) -> ()
                  }
                }
              }
              frame True {
                n604 = local read "Sweep Rate (T/min)"() -> (w1169:dbl)
                n605 = call "ips_switchHeaterOff.vi"("Instrument address"=w1170, "Rate"=w1169) -> ("B"=w1168:dbl)
                n606 = local write "Nominal Field (T)"(w1168) -> ()
              }
            }
          }
        }
      }
      event "Go to Set": Value Change {
        n607 = event-data() -> ()  [unwired: 1 in, 6 out]
        n608 = local read "Lock_in_Amplifier"() -> (w1173:refnum<visa-resource-name>)
        n609 = local read "Sweep Rate (T/min)"() -> (w1175:dbl)
        n610 = local read "Magnet"() -> (w1176:bool)
        n611 = call "Ramp_Field.vi"("Set Field (T) in"="Set Field (T)", "Sweep Rate (T/min)"=w1175, "error in (no error)"=w1177, "Magnet"=w1176, "VISA Refnum in"=w1173) -> ("error out"=w1179:errorcluster, "Actual Voltage (V)"=w1171:dbl, "Set Field (T) out"=w1174:dbl)  [unwired: 4 in]
        n612 = local write "Actual B Field (T)"(w1174) -> ()
        n613 = local write "Hall Resistance (Ohm)"(w1171) -> ()
      }
      event "Measure /Pause": Value Change {
        n614 = event-data() -> ("NewVal"=w1181:bool)  [unwired: 1 in, 5 out]
        n615 = local write "Measuring"(w1181) -> ()
      }
      event "Stop": Value Change {
        n616 = event-data() -> ()  [unwired: 1 in, 6 out]
        n617 = local read "Measuring"() -> (w1189:bool)
        n618 = case shown="True" w1189 {
          tunnel: w1188 -> [w1190 w1193]
          tunnel: [w1190 w1194] -> w1187
          frame False {
          }
          frame True {
            w1199 = FALSE ("Measuring")
            n619 = local read "SaveSweep"() -> (w1200:bool)
            n620 = local write "Measuring"(w1199) -> ()
            n621 = local write "Measure /Pause"(w1199) -> ()
            n622 = local read "Lock_in_Amplifier"() -> (w1195:refnum<visa-resource-name>)
            n623 = case shown="True" w1200 {
              frame False {
              }
              frame True {
                w1206 = 1 ("index (row)")
                w1207 = 0 ("index (row)")
                n624 = local read "Measurement File_average"() -> (w1219:path)
                n625 = local read "Averaged P(B)"() -> (w1208:dbl[][])
                n626 = local read "Averaged dt"() -> (w1210:dbl[][])
                n627 = local read "I(B) /Averaged/"() -> (w1218:cluster{"B array":dbl[], dbl[]}[])
                n628 = Index Array(array=w1210, index (row)=w1207) -> (element=w1209:dbl[])  [unwired: 1 in]
                n629 = Index Array(array=w1210, index (row)=w1206) -> (element=w1202:dbl[])  [unwired: 1 in]
                n630 = Index Array(array=w1218, index=1) -> (element=w1214:cluster{"B array":dbl[], dbl[]})
                n631 = Index Array(array=w1218, index=0) -> (element=w1215:cluster{"B array":dbl[], dbl[]})
                n632 = Unbundle(w1214) -> ("B array"=w1204:dbl[], w1203:dbl[])
                n633 = Unbundle(w1215) -> ("B array"=w1213:dbl[], w1212:dbl[])
                n634 = Index Array(array=w1208, index (row)=w1207) -> (element=w1205:dbl[])  [unwired: 1 in]
                n635 = Index Array(array=w1208, index (row)=w1206) -> (element=w1201:dbl[])  [unwired: 1 in]
                n636 = Build Array(w1213, w1212, w1209, w1205, w1204, w1203, w1202, w1201) -> (w1211:dbl[][])
                n637 = call-poly <vilib>:"Write Delimited Spreadsheet.vi"("file path (dialog if empty)"=w1219, "format (%.3f)"="%.5g", "2D data"=w1211, "append to file? (F)"=TRUE ("transpose? (F)"), "transpose? (F)"=TRUE ("append to file? (F)")) -> ()  [unwired: 9 in, 2 out]
              }
            }
            n638 = local read "Sweep Rate (T/min)"() -> (w1197:dbl)
            n639 = local read "Set Field (T)"() -> (w1198:dbl)
            n640 = local read "Magnet"() -> (w1196:bool)
            n641 = call "Ramp_Field.vi"("Set Field (T) in"=w1198, "Sweep Rate (T/min)"=w1197, "error in (no error)"=w1193, "Magnet"=w1196, "VISA Refnum in"=w1195) -> ("error out"=w1194:errorcluster, "Actual Voltage (V)"=w1191:dbl, "Set Field (T) out"=w1192:dbl)  [unwired: 4 in]
            n642 = local write "Actual B Field (T)"(w1192) -> ()
            n643 = local write "Hall Resistance (Ohm)"(w1191) -> ()
          }
        }
      }
      event "Sweep": Value Change {
        n644 = event-data() -> ("NewVal"=w1226:bool)  [unwired: 1 in, 5 out]
        n645 = case shown="True" w1226 {
          frame False {
          }
          frame True {
            n646 = local read "Measurement File"() -> (w1227:path)
            n647 = Two Button Dialog(message="Do you want to create additional files for the sweeping measurements?" ("string"), 1:"No" ("F button name (\"Cancel\")"), 2:"Yes" ("T button name (\"OK\")")) -> (T button?=w1229:bool)
            n648 = case shown="True" w1229 {
              tunnel: w1227 -> [_ w1234]
              frame False {
                n649 = local write "SaveSweep"(FALSE ("SaveSweep")) -> ()
              }
              frame True {
                n650 = call "Create_sweep_files.vi"("Measurement File"=w1234) -> ("Path 3"=→"Measurement File_dn":path, "Path 2"=→"Measurement File_up":path, "Path"=→"Measurement File_average":path)  [unwired: 8 in]
                "SaveSweep" <- TRUE
              }
            }
          }
        }
      }
      event "Measure Noise": Value Change {
        n651 = event-data() -> ("NewVal"=w1241:bool)  [unwired: 1 in, 5 out]
        n652 = case shown="True" w1241 {
          frame False {
          }
          frame True {
            n653 = local read "Gain (V/A)"() -> (w1246:dbl)
            n654 = call "Noise_measurement.vi"("Gain (V/A)"=w1246, "Cycles"="Cycles", "Lower Cut-Off"="Cut-Off Frequency", "minimum value"="minimum value", "Filter On"="Filter On", "maximum value"="maximum value", "physical channels"="physical channels", "rate"="Rate", "samples per channel"="Samples per channel") -> ("Current (pA) Filtered"=→"Current (pA) Filtered":waveform(dbl), "PSD (pA/Hz^1/2) Peaks Removed"=→"PSD (pA/Hz^1/2) Peaks Removed":cluster{"f0":dbl, "df":dbl, "magnitude":dbl[]}, "Current (pA)"=→"Current (pA)":dbl[], "PSD (pA/Hz^1/2)"=→"PSD (pA/Hz^1/2)":cluster{"f0":dbl, "df":dbl, "magnitude":dbl[]})  [unwired: 3 in]
          }
        }
      }
      event "Calibrate": Value Change {
        n655 = event-data() -> ()  [unwired: 1 in, 6 out]
        n656 = case shown="True" "Calibrate" {
          frame False {
          }
          frame True {
            w1260 = dbl[] []
            n657 = while {
              shift-right: [w1277] -> _
              shift-left: w1260 -> [w1278]
              shift-right: [w1271] -> _
              shift-left: w1260 -> [w1272]
              shift-right: [w1274] -> _
              shift-left: "Start Field" -> [w1273]
              tunnel: [w1269] -> w1261
              stop <- w1279 stop-if-true
              n658 = call "Calibration_Hall.vi"("Dwell Time (ms)"="Dwell Time (ms)", "R array in (V)"=w1272, "Max Field"="Max Field", "B array in (T)"=w1278, "Set Field (T)"=w1273, "dB"="dB") -> ("R array out (V)"=w1271:dbl[], "Ready?"=w1281:bool, 14:"Calibration Curve"=w1269:dbl[][], 15:"Calibration Curve"=→"Calibration Curve":cluster{dbl[], dbl[]}[], "B array Out"=w1277:dbl[], "Set Field out"=w1274:dbl)  [unwired: 8 in]
              "Calibration Curve Data" <- w1269
              n659 = Or(x=w1281, y="stop 2") -> (x .or. y?=w1279:bool)
            }
            n660 = flat-sequence {
              tunnel: w1261 -> [w1264]
              frame #0 {
                n661 = Two Button Dialog(message="Do you want to save calibration file?") -> (T button?=w1263:bool)  [unwired: 2 in]
                n662 = case shown="True" w1263 {
                  tunnel: w1264 -> [_ w1267]
                  frame False {
                  }
                  frame True {
                    n663 = Transpose 2D Array(2D array=w1267) -> (transposed array=w1265:dbl[][])
                    n664 = call-poly <vilib>:"Write Delimited Spreadsheet.vi"("format (%.3f)"="%.8f", "2D data"=w1265) -> ()  [unwired: 12 in, 2 out]
                  }
                }
              }
            }
          }
        }
      }
      event "New Measurement File": Value Change {
        n665 = event-data() -> ()  [unwired: 1 in, 6 out]
        n666 = local read "Sweep"() -> (w1283:bool)
        n667 = Open/Create/Replace File(prompt="Please select measurement file\n", operation (0:open)=T5."replace or create with confirmation") -> (refnum out=w1289:refnum<file>)  [unwired: 4 in, 2 out]
        n668 = local write "refnum out"(w1289) -> ()
        n669 = Refnum to Path(1:w1289) -> (0:w1284:path)
        n670 = case shown="True" w1283 {
          tunnel: w1284 -> [_ w1292]
          frame False {
          }
          frame True {
            n671 = Two Button Dialog(message="Do you want to create additional files for the sweeping measurements?" ("string"), 1:"No" ("F button name (\"Cancel\")"), 2:"Yes" ("T button name (\"OK\")")) -> (T button?=w1294:bool)
            n672 = case shown="True" w1294 {
              tunnel: w1292 -> [_ w1302]
              frame False {
                n673 = local write "SaveSweep"(FALSE ("SaveSweep")) -> ()
              }
              frame True {
                n674 = call "Create_sweep_files.vi"("Measurement File"=w1302) -> ("Path 3"=w1299:path, "Path 2"=w1300:path, "Path"=w1301:path)  [unwired: 8 in]
                n675 = local write "Measurement File_dn"(w1299) -> ()
                n676 = local write "Measurement File_average"(w1301) -> ()
                n677 = local write "Measurement File_up"(w1300) -> ()
                n678 = local write "SaveSweep"(TRUE) -> ()
              }
            }
          }
        }
        n679 = local write "Measurement File"(w1284) -> ()
        n680 = local write "Offset?"(FALSE ("Offset?")) -> ()
        n681 = local write "First?"(TRUE ("First?")) -> ()
      }
      event "Heater On/Off": Value Change {
        n682 = event-data() -> ()  [unwired: 1 in, 6 out]
        n683 = case shown="True" "Heater On/Off" {
          tunnel: w1307 -> [w1317 w1327]
          tunnel: w1306 -> [w1316 w1328]
          tunnel: [w1315 w1326] -> w1305
          frame False {
            n684 = local read "Heater 2/1"() -> (w1309:bool)
            n685 = Select(t="1,0  " ("write buffer"), s=w1309, f="2,0 " ("write buffer")) -> (s? t:f=w1310:string)
            n686 = Concatenate Strings("RANGE," ("write buffer"), w1310) -> (w1312:string)
            n687 = VISA Write(VISA resource name=w1317, write buffer=w1312, error in (no error)=w1316) -> (error out=w1315:errorcluster)  [unwired: 2 out]
          }
          frame True {
            n688 = Number To Decimal String(number="Heater Range") -> (decimal integer string=w1320:string)  [unwired: 1 in]
            n689 = local read "Heater 2/1"() -> (w1318:bool)
            n690 = Select(t="1,  " ("write buffer"), s=w1318, f="2,  " ("write buffer")) -> (s? t:f=w1319:string)
            n691 = Concatenate Strings("RANGE," ("write buffer"), w1319, w1320) -> (w1323:string)
            n692 = VISA Write(VISA resource name=w1327, write buffer=w1323, error in (no error)=w1328) -> (error out=w1326:errorcluster)  [unwired: 2 out]
          }
        }
      }
      event "Set temperature (K)": Value Change {
        n693 = event-data() -> ()  [unwired: 1 in, 6 out]
        n694 = local read "Set temperature (K)"() -> (w1339:dbl)
        n695 = local read "Heater 2/1"() -> (w1329:bool)
        n696 = Number To Fractional String(number=w1339, precision (6)=i16 3) -> (F-format string=w1342:string)  [unwired: 2 in]
        n697 = Select(t="1,  " ("write buffer"), s=w1329, f="2,  " ("write buffer")) -> (s? t:f=w1330:string)
        n698 = Concatenate Strings("SETP " ("write buffer"), w1330, w1342) -> (w1340:string)
        "concatenated string" <- w1340
        n699 = VISA Write(VISA resource name=w1336, write buffer=w1340, error in (no error)=w1338) -> (error out=w1337:errorcluster)  [unwired: 2 out]
        "error out 2" <- w1337
      }
      event "Temp Ramping Rate (K/min)": Value Change {
        n700 = event-data() -> ()  [unwired: 1 in, 6 out]
        n701 = local read "Heater 2/1"() -> (w1343:bool)
        n702 = local read "Temp Ramping Rate (K/min)"() -> (w1351:dbl)
        n703 = Number To Fractional String(number=w1351, precision (6)=i16 1) -> (F-format string=w1348:string)  [unwired: 2 in]
        n704 = Select(t="1,1,  " ("write buffer"), s=w1343, f="2,1,  " ("write buffer")) -> (s? t:f=w1344:string)
        n705 = Concatenate Strings("RAMP " ("string"), w1344, w1348) -> (w1355:string)
        n706 = VISA Write(VISA resource name=w1354, write buffer=w1355, error in (no error)=w1353) -> (error out=w1352:errorcluster)  [unwired: 2 out]
      }
      event "Heater Range": Value Change {
        n707 = event-data() -> ()  [unwired: 1 in, 6 out]
        n708 = local read "Heater On/Off"() -> (w1361:bool)
        n709 = case shown="True" w1361 {
          tunnel: w1360 -> [w1362 w1372]
          tunnel: [w1362 w1371] -> w1359
          tunnel: w1357 -> [_ w1370]
          frame False {
          }
          frame True {
            n710 = local read "Heater Range"() -> (w1368:enum16{"Off", "Low", "Medium", "High"})
            n711 = Number To Decimal String(number=w1368) -> (decimal integer string=w1367:string)  [unwired: 1 in]
            n712 = local read "Heater 2/1"() -> (w1363:bool)
            n713 = Select(t="1,  " ("write buffer"), s=w1363, f="2,  " ("write buffer")) -> (s? t:f=w1364:string)
            n714 = Concatenate Strings("RANGE," ("write buffer"), w1364, w1367) -> (w1373:string)
            n715 = VISA Write(VISA resource name=w1370, write buffer=w1373, error in (no error)=w1372) -> (error out=w1371:errorcluster)  [unwired: 2 out]
          }
        }
      }
    }
    n716 = Reciprocal(x="Sampling rate (Hz)") -> (1/x=w1017:dbl)
    n717 = Multiply(x=w1017, y=1000.0) -> (x*y=w1015:dbl)
    n718 = Wait Until Next ms Multiple(millisecond multiple=w1015) -> ()  [unwired: 1 out]
  }
  n719 = local read "Max Field (T)"() -> (w85:dbl)
  n720 = local read "Min Field (T)"() -> (w87:dbl)
  n721 = local read "dB (T)"() -> (w86:dbl)
  n722 = Divide(x=w85, y=w86) -> (x/y=w88:dbl)
  n723 = for {
    N: w88 -> [_]
    tunnel: w86 -> [w1378]
    tunnel: [w1375] -> w51 mode=indexing
    tunnel: w87 -> [w1376]
    tunnel: [0.0] -> _ mode=indexing
    i -> [w1379]
    n724 = Multiply(x=w1379, y=w1378) -> (x*y=w1377:dbl)
    n725 = Add(x=w1377, y=w1376) -> (x+y=w1375:dbl)
  }
  n726 = Multiply(x=w51, y=0.0) -> (x*y=w48:dbl[])
  n727 = Array Size(array=w48) -> (size(s)=w47:i32)
  n728 = Decrement(x=w47) -> (x-1=w46:i32)
  n729 = local write "B array"(w51) -> ()
  n730 = Array Subset(array=w48, length=w46) -> (w45:dbl[])  [unwired: 1 in]
  n731 = Build Array(w48, w48) -> (w49:dbl[][])
  n732 = local read "Max temperature (K)"() -> (w17:dbl)
  n733 = local read "Min Temperature (K)"() -> (w19:dbl)
  n734 = local write "Averaged I(B)"(w49) -> ()
  n735 = Build Array(w45, w45) -> (w44:dbl[][])
  n736 = Divide(x=w17, y="dt (K)") -> (x/y=w21:dbl)
  n737 = local write "Averaged P(B)"(w44) -> ()
  n738 = local write "Averaged dt"(w44) -> ()
  n739 = for {
    N: w21 -> [_]
    tunnel: "dt (K)" -> [w1384]
    tunnel: [w1381] -> w20 mode=indexing
    tunnel: w19 -> [w1382]
    tunnel: [0.0] -> _ mode=indexing
    i -> [w1385]
    n740 = Multiply(x=w1385, y=w1384) -> (x*y=w1383:dbl)
    n741 = Add(x=w1383, y=w1382) -> (x+y=w1381:dbl)
  }
  "T array" <- w20
  n742 = local read "Lake Shore"() -> (w98:refnum<visa-resource-name>)
  n743 = local read "IV converter"() -> (w113:refnum<visa-resource-name>)
  n744 = local read "Magnetic Field"() -> (w112:refnum<visa-resource-name>)
  n745 = VISA Close(VISA resource name=w113, error in (no error)=w115) -> (error out=w116:errorcluster)
  n746 = VISA Close(VISA resource name=w112, error in (no error)=w116) -> (error out=w114:errorcluster)
  n747 = Release Queue(queue=w120, error in (no error)=w114) -> (error out=w110:errorcluster)  [unwired: 1 in, 2 out]
  n748 = Merge Errors(w110, w7) -> (w111:errorcluster)
  n749 = VISA Close(VISA resource name=w98, error in (no error)=w111) -> (error out=w109:errorcluster)
  n750 = local read "refnum out"() -> (w107:refnum<file>)
  n751 = Close File(refnum=w107, error in=w109) -> (error out=w108:errorcluster)  [unwired: 1 out]
  n752 = call <vilib>:"Simple Error Handler.vi"("error in (no error)"=w108) -> ()  [unwired: 4 in, 5 out]
  "i" <- w78
  "j" <- w78
